vi "Old Master Control Loops.vi"() -> ()   [LabVIEW 2009]
uses:
  lib/DAQ IO/Daq Actions.ctl
  lib/Data Access Objects/Metadata/LBCB Number.ctl
  lib/Control Loop/Parameters Changes.ctl
  lib/Data Access Objects/Metadata/Persistant DAO Actions.ctl
  lib/MixedMode/Mixed Mode States.ctl
  lib/MixedMode/Ramp Time Tuple.ctl
  lib/Data Access Objects/Metadata/LBCB Filter.ctl
  lib/MixedMode/Mixed Mode Command Action.ctl
  lib/MixedMode/Mixed Mode Covergance Status.ctl
  lib/MixedMode/Mixed Mode Cartesian Data.ctl
  lib/MixedMode/Target Data.ctl
  lib/MixedMode/Messages/Mixed Mode Command.ctl
  lib/Data Access Objects/Metadata/LBCB Space.ctl
  lib/Global Data/Cartesian Data type.ctl
  lib/Global Data/Actuator DataType.ctl
  lib/Global Data/Actuator Measurment Actions.ctl
  lib/Global Data/Cartesian Measurment Actions.ctl
  lib/Control Loop/Control Loop State.ctl
  lib/Data Access Objects/Metadata/DAO Actions.ctl
  lib/Control Loop/Parameter Change States.ctl
  lib/MixedMode/Messages/Mixed Mode Status.ctl
  lib/Apps/App Status Actions.ctl
  lib/Logging/LogFileType.ctl
  lib/Launcher/Launcher Actions.ctl
  lib/Launcher/NoPanelAppTypes.ctl
  lib/Autobalance/Autobalance State.ctl
  lib/Apps/Yes No Button.ctl
  lib/Control Loop/Limit Settings.ctl
  lib/Control Loop/Limit Matrix.ctl
  lib/Control Loop/LBCB_Conversions_Actions.ctl
  lib/Data Access Objects/Global Cache/Global Cache.vi
  lib/Data Access Objects/Metadata/LBCB Settings.ctl
  lib/Data Access Objects/Control Loop/PID Controls.ctl
  lib/MixedMode/Stiffness Matrix.ctl
  lib/Data Access Objects/Metadata/LBCB Position.ctl
  lib/Limits/Actuator Faults.ctl
  lib/Limits/Cart Force Faults.ctl
  lib/Limits/Cart Disp Faults.ctl
  lib/Data Access Objects/Metadata/LBCB Size.ctl
  lib/Data Access Objects/Metadata/LBCB Type.ctl
  lib/Control Loop/Act & Cart Measurments.ctl
  lib/Autobalance/Autobalance Status Data.ctl
  lib/Control Loop/Act & Cart Commands.ctl
  lib/Autobalance/Autobalance Stage.ctl
  lib/Autobalance/Autobalance Data Point.ctl
panel:
  in  "Monitor Loop Time":u32
  out "L2 Volts LVDT & LC":dbl[](array[numeric])
  out "L1 Volts LVDT & LC":dbl[](array[numeric])
  out "L2 Autobalance Out":T1[](array[typedef])
  out "L1 Autobalance Out":T1[](array[typedef])
  out "Collecting DAQ Samples":bool
  out "DAQ Volts":dbl[](array[numeric])=[-5.059315779335383, -5.016629198362524, -5.097891313865665, -5.092890991738198, -5.1138932889519, -4.974194835814303, 0.24442110332308561, 0.2508540081873783, -0.00045656932832031883, -0.0010919008583725697, -0.001119467422792373, -0.001138029771633142, 0.051584220664617125, 0.05637080163747566, -0.0007913138656640637, 0.023009008261802286, -0.021593288951899364, 0.0027051641856972383, -5.059665406563526, -5.018353952939143, -5.097893414204858, -5.0928919356893525, -5.11389113151188, -4.974191443340161, 0.24267296718237016, 0.2422302353042843, -0.0004670710242903981, -0.0011032282722249686, -0.0010935781425555466, -0.0010973200819313358, 0.05123459343647403, 0.05464604706085686, -0.0007934142048580796, 0.02300806431064792, -0.02159113151187963, 0.0027085566598390553, 0.048884220664617124, 0.04853459343647403, 0.050170801637475664, 0.04844604706085686, -9.131386566406377e-05, -9.341420485807962e-05]
  in  "Volt Logger Time":u32
  out "All Stopped":bool
  out "L2 Previous Target":T5
  out "L1 Previous Target":T5
  out "L2 Iterative Target":T6
  out "L1 Iterative Target":T6
  out "Mixed Mode":i32
  out "Status Changes":i32
  out "L2 Control Rate":i32
  out "DAQ Started":bool
  out "L2 Current Target":T6
  out "L1 Current Target":T6
  out "Logging Directory":path
  out "L2 Auto Balance Error Tolerance":dbl[](array[numeric])=[0.01, 0.01, 0.01, 0.01, 0.01, 0.01]
  out "L1 Auto Balance Error Tolerance":dbl[](array[numeric])=[0.01, 0.01, 0.01, 0.01, 0.01, 0.01]
  out "L2 PID Control":T8={"I-Control"=TRUE, "Ctrl Mode"=TRUE}
  in  "Hold Period":bool
  in  "Averaging":bool
  out "L1 Ctrl Loop State":T9
  out "L2 Max Increment":dbl[](array[numeric])
  out "L2 Jacobian Gain":dbl[](array[numeric])
  out "L2 Force Error Range":dbl[](array[numeric])
  out "L1 Max Increment":dbl[](array[numeric])
  out "L1 Jacobian Gain":dbl[](array[numeric])
  out "L1 Force Error Range":dbl[](array[numeric])
  out "L2 Commands":T10
  out "L1 Commands":T10
  out "L2 I Gain":dbl[](array[numeric])=[0.3, 0.3, 0.3, 0.3, 0.3, 0.3]
  in  "L2 PID On":bool
  in  "L2 Faults":T14
  in  "L2 Ctrl Loop In Actuator":dbl[](array[numeric])
  out "L2 Cmd  Volts":dbl[](array[numeric])
  out "L2 Ctrl Loop Out Actuator":dbl[](array[numeric])=[0.012801822908652838, 0.012801822908652838, 7.98290599846041e-06, 8.154359441903125e-06, 8.154359441903125e-06, 8.154359441903125e-06]
  out "L2 P Gain":dbl[](array[numeric])
  out "L2 I Const":dbl[](array[numeric])
  in  "Ramp Time":u32
  out "LBCB 2 Setting":T15={"Size"=enum."1/5th-scale LBCB", "Type"=enum."Left Hand Type"}
  out "L2 Limits":T18
  out "L1  Limits":T18
  out "L2 Position":T20={"Motion Center"=[0.0, 0.0, 0.0], "Transformation Matrix"=[[1.0, 0.0, 0.0, 0.0, 0.0, 0.0], [0.0, 1.0, 0.0, 0.0, 0.0, 0.0], [0.0, 0.0, 1.0, 0.0, 0.0, 0.0], [0.0, 0.0, 0.0, 1.0, 0.0, 0.0], [0.0, 0.0, 0.0, 0.0, 1.0, 0.0], [0.0, 0.0, 0.0, 0.0, 0.0, 1.0]]}
  out "L1  Position":T20={"Motion Center"=[0.0, 0.0, 0.0], "Transformation Matrix"=[[1.0, 0.0, 0.0, 0.0, 0.0, 0.0], [0.0, 1.0, 0.0, 0.0, 0.0, 0.0], [0.0, 0.0, 1.0, 0.0, 0.0, 0.0], [0.0, 0.0, 0.0, 1.0, 0.0, 0.0], [0.0, 0.0, 0.0, 0.0, 1.0, 0.0], [0.0, 0.0, 0.0, 0.0, 0.0, 1.0]]}
  out "L1 Measurements":T21
  out "L2 Measurements":T21
  out "L1 Stiffness Jacobian":T22=[[1000000.0, 0.0, 0.0, 0.0, 0.0, 0.0], [0.0, 1000000.0, 0.0, 0.0, 0.0, 0.0], [0.0, 0.0, 1000000.0, 0.0, 0.0, 0.0], [0.0, 0.0, 0.0, 1000000.0, 0.0, 0.0], [0.0, 0.0, 0.0, 0.0, 1000000.0, 0.0], [0.0, 0.0, 0.0, 0.0, 0.0, 1000000.0]]
  out "L2 Stiffness Jacobian":T22=[[1000000.0, 0.0, 0.0, 0.0, 0.0, 0.0], [0.0, 1000000.0, 0.0, 0.0, 0.0, 0.0], [0.0, 0.0, 1000000.0, 0.0, 0.0, 0.0], [0.0, 0.0, 0.0, 1000000.0, 0.0, 0.0], [0.0, 0.0, 0.0, 0.0, 1000000.0, 0.0], [0.0, 0.0, 0.0, 0.0, 0.0, 1000000.0]]
  out "L1 Convergence Status":T23
  out "L2 Convergence Status":T23
  out "MixedModeStates":T24
  out "L1 PID Control":T8={"I-Control"=TRUE, "Ctrl Mode"=TRUE}
  in  "L1 PID On":bool
  in  "L1 Faults":T14
  out "L1 P Gain":dbl[](array[numeric])
  out "L1 I Gain":dbl[](array[numeric])=[0.3, 0.3, 0.3, 0.3, 0.3, 0.3]
  out "L1 I Const":dbl[](array[numeric])
  out "LBCB 1 Control Loop Force Limit":bool
  out "LBCB 1 Setting":T15={"Size"=enum."1/5th-scale LBCB", "Type"=enum."Left Hand Type"}
  out "L2 Ctrl Loop State":T9
  out "L1 Cmd  Volts":dbl[](array[numeric])
  out "L1 Ctrl Loop Out Actuator":dbl[](array[numeric])=[0.012801822908652838, 0.012801822908652838, 7.98290599846041e-06, 8.154359441903125e-06, 8.154359441903125e-06, 8.154359441903125e-06]
  out "L1 Control Rate":i32=50 caption="Control Rate"
  in  "L1 Ctrl Loop In Actuator":dbl[](array[numeric])
  out "L2 Servo Error":dbl[](array[numeric])=[-0.014471871278962644, -0.0027477897622864888, 0.03594582291831433, -0.006177356244415369, -0.000527948512754489, 0.04718526152757189]
  out "L2 Actuator Meas. Disp & Forces":dbl[](array[numeric])=[0.015224103858920254, 0.016374115079328375, 0.0001743188568230551, 0.03971045114557009, 0.007082336209989981, 0.009859079687370698, 8.685887933911959, 1.9897804119684945, 4.857688782335148, 93.30834661628205, -5.911514458784602, -1.446477360303783]
  out "Number of \nExternal \nChannels":i32
  out "DAQ Enabled":bool
  in  "App Running":bool
  out "DAQ Rate":i32=2 caption="Control Rate"
  out "L1 Servo Error":dbl[](array[numeric])=[-0.014471871278962644, -0.0027477897622864888, 0.03594582291831433, -0.006177356244415369, -0.000527948512754489, 0.04718526152757189]
  out "L1 Actuator Meas. Disp & Forces":dbl[](array[numeric])=[0.015224103858920254, 0.016374115079328375, 0.0001743188568230551, 0.03971045114557009, 0.007082336209989981, 0.009859079687370698, 8.685887933911959, 1.9897804119684945, 4.857688782335148, 93.30834661628205, -5.911514458784602, -1.446477360303783]
  out "External Sensors":dbl[](array[numeric])
  out "DAQ Overflow":bool
  # "Cmd"
  # "Servo"
  # "Cmd"
  # "Servo"
  # "Cmd"
  # "Servo"
  # "Cmd"
  # "Servo"
  # "Continuous"
  # "Hold"
  # "(inch)"
  # "X"
  # "(inch)"
  # "Y"
  # "(inch)"
  # "Z"
  # "Xglobal = T*Xlocal"
  # "(inch)"
  # "X"
  # "(inch)"
  # "Y"
  # "(inch)"
  # "Z"
  # "Xglobal = T*Xlocal"
  # "Continuous"
  # "Hold"
types:
  T1 = typedef "Autobalance Status Data.ctl" = cluster{"IsBalanced":T2, "Autobalance Stage":T3, "High":T4, "Low":T4, "Balanced \nCmd":dbl}
  T2 = typedef "Yes No Button.ctl" = bool
  T3 = typedef "Autobalance Stage.ctl" = enum16{"Coarse", "Fine", "Backing Up", "Done"}
  T4 = typedef "Autobalance Data Point.ctl" = cluster{"cCmd":dbl, "cServo":dbl, "pCmd":dbl, "pServo":dbl}
  T5 = typedef "Mixed Mode Cartesian Data.ctl" = cluster{"Displacements":dbl[], "Forces":dbl[]}
  T6 = typedef "Target Data.ctl" = cluster{"Displacements":dbl[], "Command Type":enum16{"<None>", "Displacement", "Force"}[], "Forces":dbl[], "Space":T7}
  T7 = typedef "LBCB Space.ctl" = enum16{"Actuator", "Cartesian"}
  T8 = typedef "PID Controls.ctl" = cluster{"I-Control":bool, "Ctrl Mode":bool}
  T9 = typedef "Control Loop State.ctl" = enum16{"Idle", "Off", "Reset Autobalancing", "Autobalancing", "Set Command", "Ready for Control", "On"}
  T10 = typedef "Act & Cart Commands.ctl" = cluster{"Act Cmd":dbl[], "Cart Cmd":dbl[]}
  T11 = typedef "Actuator Faults.ctl" = cluster{"X1":bool, "X2":bool, "Y1":bool, "Z1":bool, "Z2":bool, "Z3":bool}
  T12 = typedef "Cart Force Faults.ctl" = cluster{"Fx":bool, "Fy":bool, "Fz":bool, "Mx":bool, "My":bool, "Mz":bool}
  T13 = typedef "Cart Disp Faults.ctl" = cluster{"Dx":bool, "Dy":bool, "Dz":bool, "Rx":bool, "Ry":bool, "Rz":bool}
  T14 = cluster{"Act Disp":T11, "Act Force":T11, "Cart Force":T12, "Cart Disp":T13}
  T15 = typedef "LBCB Settings.ctl" = cluster{"Size":T16, "Type":T17}
  T16 = typedef "LBCB Size.ctl" = enum16{"1/5th-scale LBCB", "Full-scale LBCB", "Portable LBCB"}
  T17 = typedef "LBCB Type.ctl" = enum16{"Right Hand Type", "Left Hand Type"}
  T18 = typedef "Limit Settings.ctl" = cluster{"Actuator Force Limits":T19, "Actuator Stroke Limits":T19, "Cartesian Disp Limit":T19, "Cartesian Force Limit":T19, "Command Voltage Limit":T19}
  T19 = typedef "Limit Matrix.ctl" = dbl[][]
  T20 = typedef "LBCB Position.ctl" = cluster{"Motion Center":dbl[], "Transformation Matrix":dbl[][]}
  T21 = typedef "Act & Cart Measurments.ctl" = cluster{"Act Disp":dbl[], "Act Forces":dbl[], "Cart Disp":dbl[], "Cart Forces":dbl[]}
  T22 = typedef "Stiffness Matrix.ctl" = dbl[][]
  T23 = typedef "Mixed Mode Covergance Status.ctl" = cluster{"IsConverged":bool[], "Force Errors":dbl[], "MaxForceDiffIndex":i32}
  T24 = typedef "Mixed Mode States.ctl" = enum16{"Init", "Wait For DAQ", "Idle", "Start Initial Position", "Initial Position", "Start Initial Ramp", "Run Initial Ramp", "Start Iterative Stage", "Convergence Check", "Update Stiffness Jacobian", "Update Command", "Start Iterative Ramp", "Run Iterative Ramp", "Start Iterative Stabilize", "Iterative Stabilize", "Start Iterative Holding", "Iterative Holding", "Start Stabilize", "Stabilize", "Start Hold", "Holding", "Done", "Aborting", "Exit", "Nop"}
  T25 = typedef "Persistant DAO Actions.ctl" = enum16{"Init", "Get", "Set", "Load", "Save"}
  T26 = typedef "Autobalance State.ctl" = enum16{"Init", "Send High ", "Wait High", "Read High Start", "Read High", "Send Low", "Wait Low", "Read Low Start", "Read Low", "Publish", "Calculate", "Done"}
  T27 = typedef "Ramp Time Tuple.ctl" = cluster{"Ramp":dbl, "Stab":dbl, "Hold":dbl}
  T28 = typedef "Mixed Mode Command Action.ctl" = enum16{"Start Command", "Stop", "Exit", "No Op", "Start Acquisition", "Measure Initial Position"}
  T29 = typedef "LBCB Number.ctl" = enum16{"LBCB1", "LBCB2"}
  T30 = typedef "Mixed Mode Status.ctl" = cluster{"LBCB Target":T6[], "MixedModeStates":T24, "LBCB Convergence":T23[], "LBCB Measurements":T5[]}
  T31 = typedef "Mixed Mode Command.ctl" = cluster{"Command":T28, "Ramp Times":cluster{"Initial":T27, "Iterative":T27}, "LBCB1":T6, "LBCB2":T6}
  T32 = typedef "Parameters Changes.ctl" = cluster{"Change State":T33, "LBCB Number":T29}
  T33 = typedef "Parameter Change States.ctl" = enum16{"Mixed Mode", "Control Loop", "Limits", "Application", "Stiffness Jacobian", "Start DAQ", "Auto-Balancing", "Set Command", "Enable Control", "Disable Control", "Stop Application"}
  T34 = typedef "Cartesian Point.ctl" = cluster{"Dx":dbl, "Dy":dbl, "Dz":dbl, "Rx":dbl, "Ry":dbl, "Rz":dbl}
  T35 = typedef "Actuator Matrix.ctl" = cluster{"Lower":T36, "Upper":T36}
  T36 = typedef "Actuator Point.ctl" = cluster{"X1":dbl, "X2":dbl, "Y1":dbl, "Z1":dbl, "Z2":dbl, "Z3":dbl}
  T37 = typedef "Cartesian Matrix.ctl" = cluster{"Lower":T34, "Upper":T34}
  T38 = typedef "App Parameters.ctl" = cluster{"Monitor Loop":T39, "Ramp Time":T39, "Log Loop":T39, "TCP to DAQ":T39, "Logging Directory":path, "Log File Size (MBytes)":i64, "Volt Logging Loop":T39}
  T39 = typedef "Timing Parameters.ctl" = cluster{"Interval":dbl, "Rate ":dbl}
  T40 = typedef "Number Of LBCBs.ctl" = enum16{"1", "2"}
  T41 = typedef "DAO Actions.ctl" = enum16{"Init", "Get", "Set"}
  T42 = typedef "Actuator Measurment Actions.ctl" = enum16{"Set  Data", "Get", "Init"}
  T43 = typedef "Actuator DataType.ctl" = cluster{"LVDTs":dbl[], " Commands":dbl[], "Load Cells":dbl[], "Servo":dbl[]}
  T44 = typedef "Cartesian Data type.ctl" = cluster{"Displacements":dbl[], "Forces":dbl[], "Displacement Commands":dbl[]}
  T45 = typedef "Cartesian Measurment Actions.ctl" = enum16{"Set Data", "Get", "Init", "Set Offsets"}
  T46 = typedef "Calibration Settings.ctl" = cluster{"Command Sensitivity":dbl[], "Servo Error Offset":dbl[], "LVDT Sensitivity":dbl[], "LVDT Offset":dbl[], "Load Cell Offsets":dbl[], "Load Cell Sensitivity":dbl[]}
  T47 = typedef "Autobalance Control Parameters.ctl" = cluster{"Number of Samples":i32, "Delay After Cmd":i32, "Maximum Command":dbl}
  T48 = typedef "App Status Actions.ctl" = enum16{"Init", "Get Status", "Running", "Control", "Autobalanced", "Data Acquisition", "Set App State", "DAQ Started", "Set LBCB State", "Set All", "Set Cont Logging", "Set Step Logging", "Set MM Logging", "Set Volt Logging", "Set Cart Type", "Set DAQ Link", "Set NTCP Link"}
  T49 = typedef "Ramp Time Input.ctl" = cluster{"Directional":T50, "Iterative":T50}
  T50 = typedef "Ramp Control.ctl" = cluster{"Ramp":dbl, "Stabilize":dbl, "Hold":dbl}
  T51 = typedef "App Status.ctl" = cluster{"Running":bool, "Controlling L2":bool, "Autobalance L2":bool, "Data Acquisition":bool, " App State":T52, "DAQ Started":bool, "LBCB 1 State":T53, "LBCB 2 State":T53, "Controlling L1":bool, "Autobalance L1":bool, "Cartesian Type":bool, "Continuous Logging":bool, "Step Logging":bool, "Voltage Logging":bool, "Mixed Mode Logging":bool, "DAQ Link":bool, "NTCP Link ":bool}
  T52 = typedef "AppStates.ctl" = enum16{"Starting OM", "Initializing Displays", "Setting up Archiving", "Setting Up DAQ Channels", "Start DAQ", "DAQ Starting", "Controlling LBCBs", "Stopping OM"}
  T53 = typedef "Lbcb Control Loop States.ctl" = enum16{"Idle", "Start Selected", "Load Last Command", "Start Autobalancing", "Autobalancing", "Control Loop Initialized", "Control Enabled"}
  T54 = typedef "LBCB_Conversions_Actions.ctl" = enum16{"A2C", "C2A", "Set Log Filename", "Init"}
  T55 = cluster{"Act Disp":dbl[], "Act Forces":dbl[], "Cart Disp":dbl[], "Cart Forces":dbl[]}
  T56 = typedef "Measurements.ctl" = cluster{"Act Disp":dbl[], "Act Forces":dbl[], "Cart Disp":dbl[], "Cart Forces":dbl[]}
  T57 = typedef "Daq Actions.ctl" = enum16{"Init", "Send Commands", "Get Responses", "Stop"}
  T58 = enum16{"open", "replace", "create", "open or create", "replace or create", "replace or create with confirmation"}
  T59 = typedef "LogFileType.ctl" = enum16{"Continuous", "Step", "Volts", "Offsets", "Mixed Mode State", "DLL  Errors", "End List"}
  T60 = typedef "LBCB Filter.ctl" = enum16{"LBCB 1", "LBCB 2", "Both"}
  T61 = typedef "NoPanelAppTypes.ctl" = enum16{"NTCP Socket", "Data Archiving", "DAQ Link", "Control Loops", "Autobalance Monitor", "Mixed Mode Monitor", "Cmd Disp Diffs"}
  T62 = typedef "Launcher Actions.ctl" = enum16{"Launch", "Stop All", "Stop", "Kill", "Running?", "Init"}
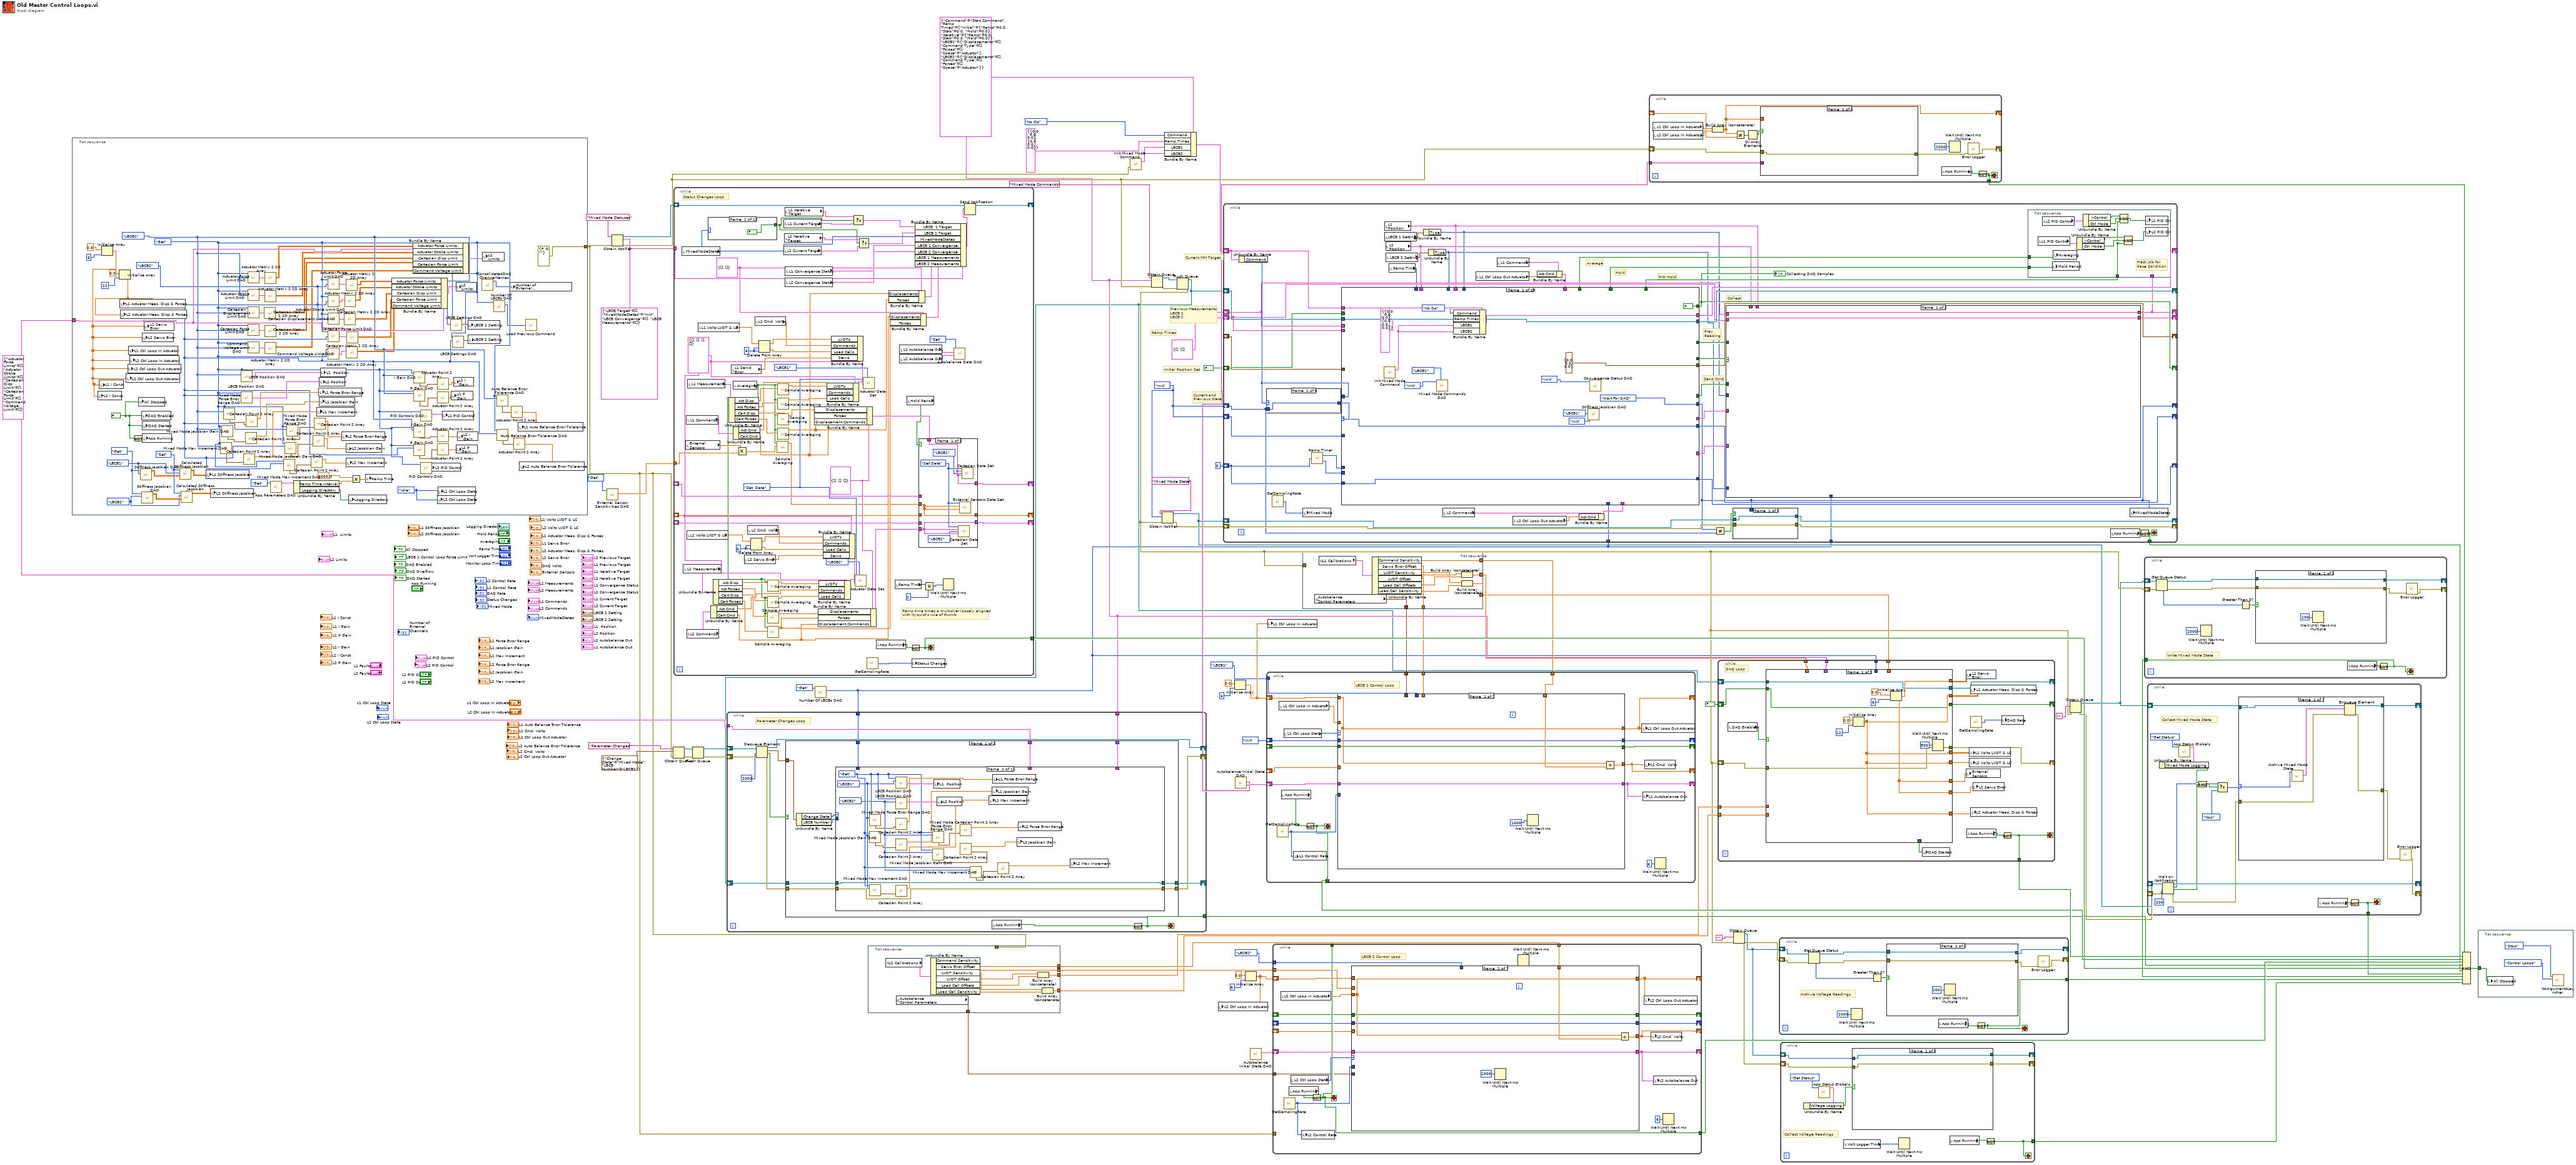
[diagram p0: block diagram]
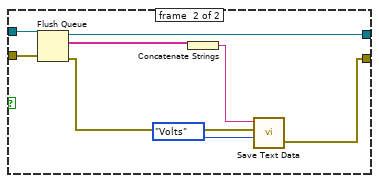
[diagram p2: hidden frame]
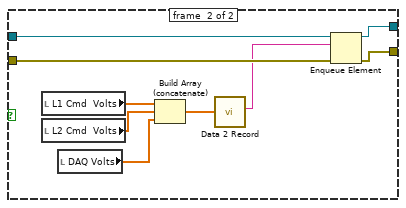
[diagram p3: hidden frame]
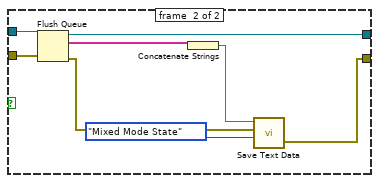
[diagram p4: hidden frame]
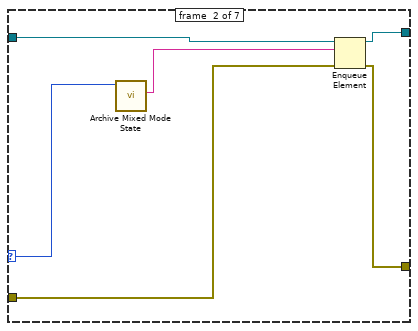
[diagram p5: hidden frame]
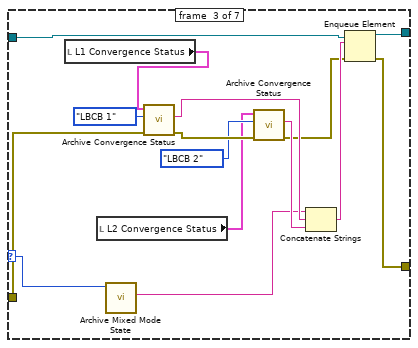
[diagram p6: hidden frame]
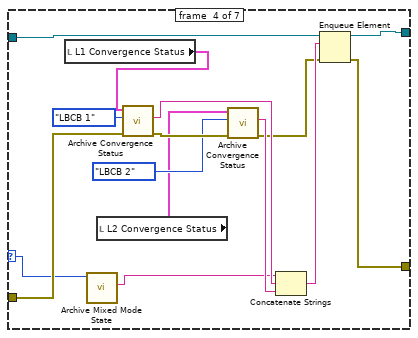
[diagram p7: hidden frame]
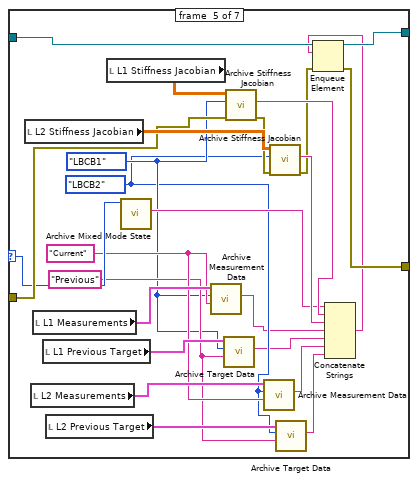
[diagram p8: hidden frame]
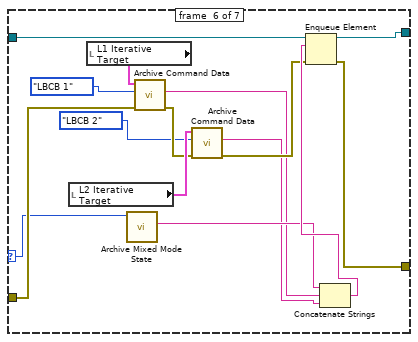
[diagram p9: hidden frame]
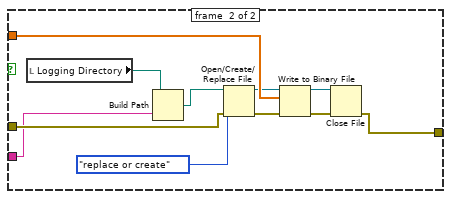
[diagram p11: hidden frame]
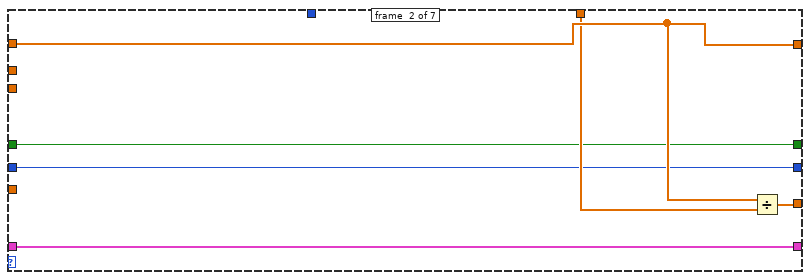
[diagram p12: hidden frame]
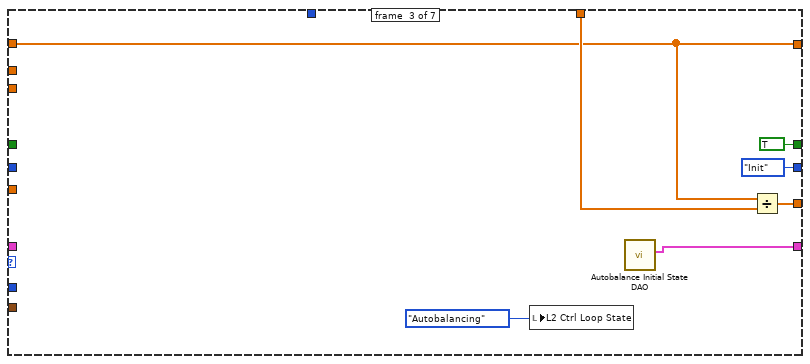
[diagram p13: hidden frame]
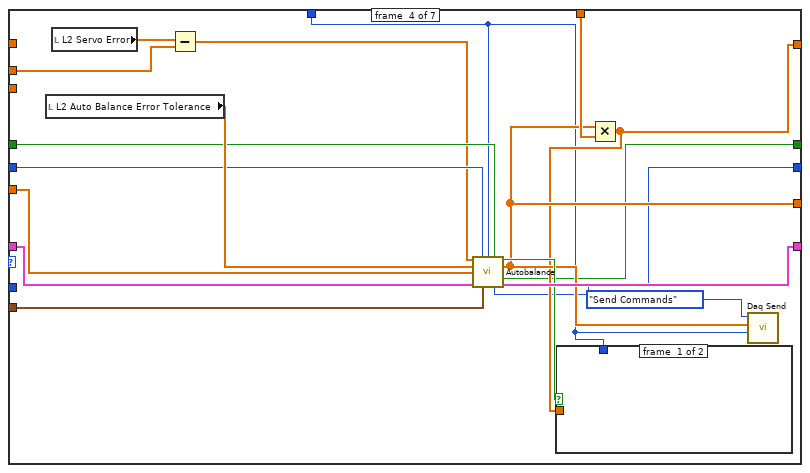
[diagram p14: hidden frame]
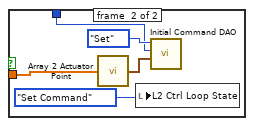
[diagram p15: hidden frame]
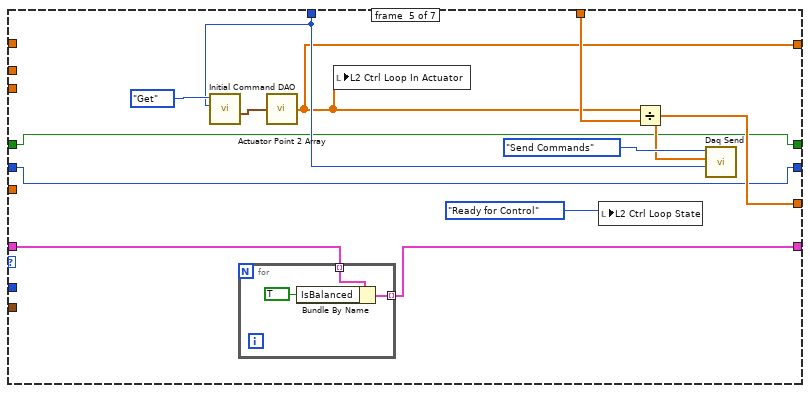
[diagram p16: hidden frame]
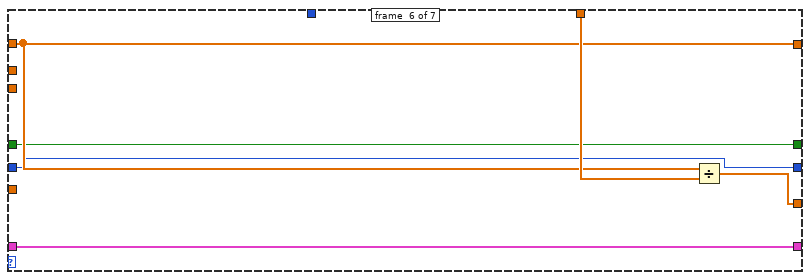
[diagram p17: hidden frame]
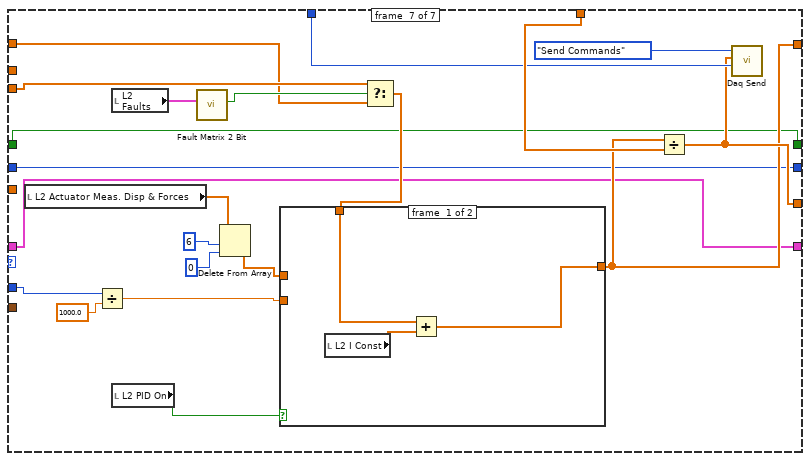
[diagram p18: hidden frame]
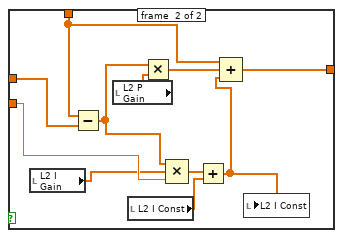
[diagram p19: hidden frame]
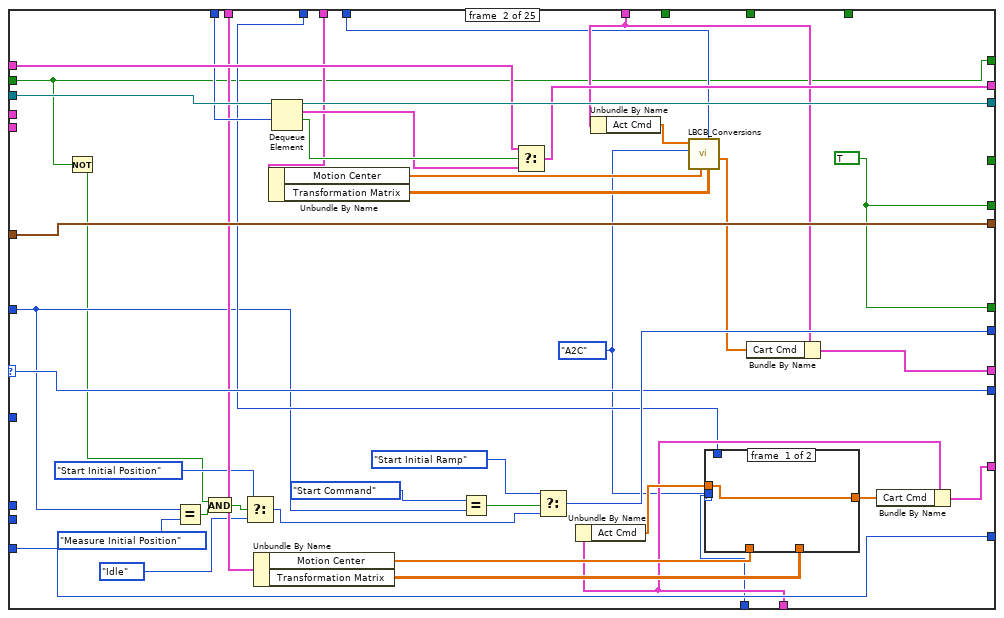
[diagram p20: hidden frame]
diagram:
  w9 = T18 {"Actuator Force Limits"=[], "Actuator Stroke Limits"=[], "Cartesian Disp Limit"=[], "Cartesian Force Limit"=[], "Command Voltage Limit"=[]} ("L1  Limits")
  w60 = T30 {"LBCB Target"=[], "MixedModeStates"=enum."Init", "LBCB Convergence"=[], "LBCB Measurements"=[]} ("Mixed Mode Status")
  w66 = T5 {"Displacements"=[], "Forces"=[]} ("Cartesian  Data")
  w3 = T31 {"Command"=enum."Start Command", "Ramp Times"={"Initial"={"Ramp"=0.0, "Stab"=0.0, "Hold"=0.0}, "Iterative"={"Ramp"=0.0, "Stab"=0.0, "Hold"=0.0}}, "LBCB1"={"Displacements"=[], "Command Type"=[], "Forces"=[], "Space"=enum."Actuator"}, "LBCB2"={"Displacements"=[], "Command Type"=[], "Forces"=[], "Space"=enum."Actuator"}} ("Mixed Mode Command")
  w70 = Mixed_Mode_States."Init" ("MixedModeStates")
  # "Initial Position Set"
  # "Current MM Target"
  # "Current and\nPrevious State"
  # "Previous Measurements\nLBCB 1\nLBCB 2"
  # "Ramp Times"
  n1 = flat-sequence {
    tunnel: [errorcluster {"status"=FALSE, "code"=0, "source"=""} ("error out")] -> w13
    tunnel: w9 -> [w95]
    frame #0 {
      w103 = Control_Loop_State."Idle" ("L1 Ctrl Loop State")
      w98 = LBCB_Number."LBCB2" ("ID")
      w100 = LBCB_Number."LBCB1" ("ID")
      w99 = Persistant_DAO_Actions."Get" ("Actuator Force Limit Actions")
      w112 = FALSE
      w138 = Persistant_DAO_Actions."Set" ("Actions")
      w135 = LBCB_Number."LBCB1" ("LBCB Number")
      w136 = LBCB_Number."LBCB2" ("LBCB Number")
      w134 = Persistant_DAO_Actions."Get" ("Actions")
      n2 = Initialize Array(0.0 ("element"), 6 ("dimension size")) -> (w102:dbl[])
      n3 = local write "L2 I Const"(w102) -> ()
      n4 = local write "L1 I Const"(w102) -> ()
      n5 = Initialize Array(0.0 ("element"), 12 ("dimension size")) -> (w104:dbl[])
      n6 = local write "L1 Actuator Meas. Disp & Forces"(w104) -> ()
      n7 = local write "L2 Actuator Meas. Disp & Forces"(w104) -> ()
      n8 = local write "L2 Ctrl Loop Out Actuator"(w102) -> ()
      n9 = local write "L1 Ctrl Loop Out Actuator"(w102) -> ()
      n10 = local write "L1 Ctrl Loop In Actuator"(w102) -> ()
      n11 = local write "L2 Ctrl Loop In Actuator"(w102) -> ()
      n12 = Not(x=w112) -> (.not. x?=w131:bool)
      n13 = local write "All Stopped"(w112) -> ()
      n14 = call "Stiffness Jacobian DAO.vi"("LBCB Number"=w135, "Actions"=w134) -> ("Stiffness Jacobian Out"=w137:T22)  [unwired: 3 in, 6 out]
      n15 = local write "DAQ Enabled"(w112) -> ()
      n16 = call "Stiffness Jacobian DAO.vi"("LBCB Number"=w136, "Actions"=w134) -> ("Stiffness Jacobian Out"=w139:T22)  [unwired: 3 in, 6 out]
      n17 = local write "L2 Servo Error"(w102) -> ()
      n18 = local write "DAQ Started"(w112) -> ()
      n19 = local write "App Running"(w131) -> ()
      n20 = local write "L1 Servo Error"(w102) -> ()
      n21 = call "Calculated Stiffness Jacobian.vi"("Stiffness Jacobian In"=w137, "LBCB Number"=w135, "Actions"=w138) -> ("Stiffness Jacobian Out"=w132:T22)  [unwired: 1 in, 7 out]
      n22 = call "Calculated Stiffness Jacobian.vi"("Stiffness Jacobian In"=w139, "LBCB Number"=w136, "Actions"=w138) -> ("Stiffness Jacobian Out"=w133:T22)  [unwired: 1 in, 7 out]
      n23 = local write "L1 Stiffness Jacobian"(w132) -> ()
      n24 = local write "L2 Stiffness Jacobian"(w133) -> ()
      n25 = call "Mixed Mode Max Increment DAO.vi"("Max Increment Actions"=w99, "LBCB Number"=w100) -> ("Max Increment Out"=w150:T34)  [unwired: 3 in, 10 out]
      n26 = call "Mixed Mode Jacobian Gain DAO.vi"("Jacobian Gain Actions"=w99, "LBCB Number"=w100) -> ("Jacobian Gain Out"=w149:T34)  [unwired: 3 in, 10 out]
      n27 = call "Mixed Mode Force Error Range DAO.vi"("Force Error Range Actions"=w99, "LBCB Number"=w100) -> ("Force Error Range Out"=w148:T34)  [unwired: 3 in, 10 out]
      n28 = call "LBCB Position DAO.vi"("LBCB Settings Actions"=w99, "LBCB Number"=w100) -> ("LBCB Position Output"=w147:T20)  [unwired: 3 in, 10 out]
      n29 = call "LBCB Position DAO.vi"("LBCB Settings Actions"=w99, "LBCB Number"=w98) -> ("LBCB Position Output"=w146:T20)  [unwired: 3 in, 10 out]
      n30 = call "Cartesian Point 2 Array.vi"("Cart Disp"=w150) -> ("Array"=w143:dbl[])  [unwired: 2 out]
      n31 = call "Cartesian Point 2 Array.vi"("Cart Disp"=w149) -> ("Array"=w144:dbl[])  [unwired: 2 out]
      n32 = call "Cartesian Point 2 Array.vi"("Cart Disp"=w148) -> ("Array"=w145:dbl[])  [unwired: 2 out]
      n33 = call "Actuator Force Limit DAO.vi"("Actuator Force Limit Actions"=w99, "ID"=w100) -> ("Actuator Force Limits Out"=w94:T35)  [unwired: 3 in, 10 out]
      n34 = call "Actuator Stroke Limit DAO.vi"("Actuator Stroke Limit Actions"=w99, "ID"=w100) -> ("Actuator Stroke Limits Out"=w93:T35)  [unwired: 3 in, 10 out]
      n35 = call "Cartesian Displacement Limit DAO.vi"("Cartesian Displacement Limit Actions"=w99, "ID"=w100) -> ("Cartesian Displacement Out"=w88:T37)  [unwired: 3 in, 10 out]
      n36 = call "Cartesian Force Limit DAO.vi"("Cartesian Force Limit Actions"=w99, "ID"=w100) -> ("Cartesian Force Limit Out"=w87:T37)  [unwired: 3 in, 10 out]
      n37 = call "Command Voltage Limit DAO.vi"("Actuator Stroke Limit Actions"=w99, "ID"=w100) -> ("Command Voltage Limit Out"=w92:T35)  [unwired: 3 in, 10 out]
      n38 = call "Cartesian Matrix 2 2D Array.vi"("Matrix In"=w88) -> ("Matrix Out"=w76:T19)  [unwired: 10 out]
      n39 = call "Actuator Matrix 2 2D Array.vi"("Matrix In"=w94) -> ("Matrix Out"=w91:T19)  [unwired: 10 out]
      n40 = call "Actuator Matrix 2 2D Array.vi"("Matrix In"=w93) -> ("Matrix Out"=w90:T19)  [unwired: 10 out]
      n41 = call "Cartesian Matrix 2 2D Array.vi"("Matrix In"=w87) -> ("Matrix Out"=w75:T19)  [unwired: 10 out]
      n42 = call "Actuator Matrix 2 2D Array.vi"("Matrix In"=w92) -> ("Matrix Out"=w89:T19)  [unwired: 10 out]
      n43 = call "App Parameters DAO.vi"("Actions"=Persistant_DAO_Actions."Get") -> ("Application Timing and Logging Out"=w154:T38)  [unwired: 3 in, 7 out]
      n44 = call "Mixed Mode Max Increment DAO.vi"("Max Increment Actions"=w99, "LBCB Number"=w98) -> ("Max Increment Out"=w111:T34)  [unwired: 3 in, 10 out]
      n45 = call "Mixed Mode Jacobian Gain DAO.vi"("Jacobian Gain Actions"=w99, "LBCB Number"=w98) -> ("Jacobian Gain Out"=w110:T34)  [unwired: 3 in, 10 out]
      n46 = call "Mixed Mode Force Error Range DAO.vi"("Force Error Range Actions"=w99, "LBCB Number"=w98) -> ("Force Error Range Out"=w109:T34)  [unwired: 3 in, 10 out]
      n47 = Unbundle By Name(w154) -> ("Ramp Time.Interval"=w155:dbl, "Logging Directory"=w151:path)
      n48 = call "Cartesian Point 2 Array.vi"("Cart Disp"=w111) -> ("Array"=w140:dbl[])  [unwired: 1 in, 1 out]
      n49 = call "Cartesian Point 2 Array.vi"("Cart Disp"=w110) -> ("Array"=w141:dbl[])  [unwired: 1 in, 1 out]
      n50 = call "Cartesian Point 2 Array.vi"("Cart Disp"=w109) -> ("Array"=w142:dbl[])  [unwired: 1 in, 1 out]
      n51 = local write "L1 Max Increment"(w143) -> ()
      n52 = local write "L1 Force Error Range"(w145) -> ()
      n53 = local write "L1 Jacobian Gain"(w144) -> ()
      n54 = local write "L2 Position"(w146) -> ()
      n55 = local write "L1  Position"(w147) -> ()
      n56 = call "Actuator Force Limit DAO.vi"("Actuator Force Limit Actions"=w99, "ID"=w98) -> ("Actuator Force Limits Out"=w86:T35)  [unwired: 3 in, 10 out]
      n57 = call "Actuator Stroke Limit DAO.vi"("Actuator Stroke Limit Actions"=w99, "ID"=w98) -> ("Actuator Stroke Limits Out"=w85:T35)  [unwired: 3 in, 10 out]
      n58 = call "Cartesian Displacement Limit DAO.vi"("Cartesian Displacement Limit Actions"=w99, "ID"=w98) -> ("Cartesian Displacement Out"=w84:T37)  [unwired: 3 in, 10 out]
      n59 = call "Cartesian Force Limit DAO.vi"("Cartesian Force Limit Actions"=w99, "ID"=w98) -> ("Cartesian Force Limit Out"=w83:T37)  [unwired: 3 in, 10 out]
      n60 = call "Command Voltage Limit DAO.vi"("Actuator Stroke Limit Actions"=w99, "ID"=w98) -> ("Command Voltage Limit Out"=w82:T35)  [unwired: 3 in, 10 out]
      n61 = local write "L2 Force Error Range"(w142) -> ()
      n62 = call "Cartesian Matrix 2 2D Array.vi"("Matrix In"=w84) -> ("Matrix Out"=w79:T19)  [unwired: 10 out]
      n63 = call "Actuator Matrix 2 2D Array.vi"("Matrix In"=w85) -> ("Matrix Out"=w80:T19)  [unwired: 10 out]
      n64 = local write "L2 Jacobian Gain"(w141) -> ()
      n65 = call "Actuator Matrix 2 2D Array.vi"("Matrix In"=w86) -> ("Matrix Out"=w81:T19)  [unwired: 10 out]
      n66 = call "Actuator Matrix 2 2D Array.vi"("Matrix In"=w82) -> ("Matrix Out"=w77:T19)  [unwired: 10 out]
      n67 = local write "L2 Max Increment"(w140) -> ()
      n68 = call "Cartesian Matrix 2 2D Array.vi"("Matrix In"=w83) -> ("Matrix Out"=w78:T19)  [unwired: 10 out]
      n69 = local write "Logging Directory"(w151) -> ()
      n70 = Multiply(x=1000.0, y=w155) -> (x*y=w152:dbl)
      n71 = local write "Ramp Time"(w152) -> ()
      n72 = Bundle By Name(cluster=w95, "Actuator Force Limits"=w81, "Actuator Stroke Limits"=w80, "Cartesian Disp Limit"=w79, "Cartesian Force Limit"=w78, "Command Voltage Limit"=w77) -> (w96:T18)
      n73 = Bundle By Name(cluster=w95, "Actuator Force Limits"=w91, "Actuator Stroke Limits"=w90, "Cartesian Disp Limit"=w76, "Cartesian Force Limit"=w75, "Command Voltage Limit"=w89) -> (w97:T18)
      n74 = call "I Gain DAO.vi"("I Gain Actions"=w99, "LBCB Number"=w100) -> ("I Gain"=w127:T36)  [unwired: 3 in, 10 out]
      n75 = call "P Gain DAO.vi"("P Gain Actions"=w99, "LBCB Number"=w100) -> ("P Gain"=w128:T36)  [unwired: 3 in, 10 out]
      n76 = call "I Gain DAO.vi"("I Gain Actions"=w99, "LBCB Number"=w98) -> ("I Gain"=w130:T36)  [unwired: 3 in, 10 out]
      n77 = call "P Gain DAO.vi"("P Gain Actions"=w99, "LBCB Number"=w98) -> ("P Gain"=w129:T36)  [unwired: 3 in, 10 out]
      n78 = call "PID Controls DAO.vi"("Actions"=w99) -> ("PID Control  Out"=w125:T8)  [unwired: 3 in, 7 out]
      n79 = call "PID Controls DAO.vi"("Actions"=w99) -> ("PID Control  Out"=w126:T8)  [unwired: 3 in, 7 out]
      n80 = local write "L2 PID Control"(w125) -> ()
      n81 = call "Actuator Point 2 Array.vi"("Actuator Point"=w127) -> ("Array"=w124:dbl[])
      n82 = call "Actuator Point 2 Array.vi"("Actuator Point"=w128) -> ("Array"=w123:dbl[])
      n83 = call "Actuator Point 2 Array.vi"("Actuator Point"=w130) -> ("Array"=w122:dbl[])
      n84 = call "Actuator Point 2 Array.vi"("Actuator Point"=w129) -> ("Array"=w121:dbl[])
      n85 = local write "L2 Ctrl Loop State"(w103) -> ()
      n86 = local write "L1 Ctrl Loop State"(w103) -> ()
      n87 = local write "L1 PID Control"(w126) -> ()
      n88 = call "LBCB Settings DAO.vi"("LBCB Number"=w100, "Actions"=w99) -> ("LBCB Setting Out"=w119:T15)  [unwired: 3 in, 6 out]
      n89 = local write "L1 P Gain"(w123) -> ()
      n90 = call "LBCB Settings DAO.vi"("LBCB Number"=w98, "Actions"=w99) -> ("LBCB Setting Out"=w118:T15)  [unwired: 3 in, 6 out]
      n91 = local write "L1 I Gain"(w124) -> ()
      n92 = local write "L2 Limits"(w96) -> ()
      n93 = local write "L2 P Gain"(w121) -> ()
      n94 = local write "L2 I Gain"(w122) -> ()
      n95 = local write "LBCB 1 Setting"(w119) -> ()
      n96 = local write "LBCB 2 Setting"(w118) -> ()
      n97 = call "ConsolidatedDAQChannelNames.vi"() -> ("Number of \nExternal \nChannels 1"=w120:i32)  [unwired: 5 out]
      n98 = local write "L1  Limits"(w97) -> ()
      n99 = call "Number Of LBCBs DAO.vi"("Actions"=w99) -> ("Number of\nLBCBs Out"=w101:T40)  [unwired: 3 in, 7 out]
      n100 = call "Auto Balance Error Tolerance DAO.vi"("Auto Balance Increment Actions"=w99, "LBCB Number"=w100) -> ("Auto Balance Error Out"=w116:T36)  [unwired: 3 in, 10 out]
      n101 = call "Auto Balance Error Tolerance DAO.vi"("Auto Balance Increment Actions"=w99, "LBCB Number"=w98) -> ("Auto Balance Error Out"=w117:T36)  [unwired: 3 in, 10 out]
      n102 = local write "Number of \nExternal \nChannels"(w120) -> ()
      n103 = call "Actuator Point 2 Array.vi"("Actuator Point"=w116) -> ("Array"=w114:dbl[])
      n104 = call "Actuator Point 2 Array.vi"("Actuator Point"=w117) -> ("Array"=w115:dbl[])
      n105 = local write "L1 Auto Balance Error Tolerance"(w114) -> ()
      n106 = local write "L2 Auto Balance Error Tolerance"(w115) -> ()
      n107 = call "Load Previous Command.vi"("Number of LBCBs"=w101) -> ()  [unwired: 3 out]
    }
  }
  n108 = call "External Sensor Sensitivities DAO.vi"("Persistent DAO Actions"=Persistant_DAO_Actions."Get") -> ("Sensitivities Out"=w16:dbl[])  [unwired: 3 in, 7 out]
  n109 = Obtain Notifier(name (unnamed)="Mixed Mode Statuses", notification data type=w60, error in (no error)=w13) -> (notifier out=w61:refnum<notifier>, error out=w15:errorcluster)  [unwired: 1 in, 1 out]
  n110 = Obtain Queue(name (unnamed)="Parameter Changes", element data type=T32 {"Change State"=enum."Mixed Mode", "LBCB Number"=enum."LBCB1"} ("Parameter Changes"), error in (no error)=w13) -> (queue out=w72:refnum<queue>, error out=w39:errorcluster)  [unwired: 2 in, 1 out]
  n111 = while {
    shift-right: [w193] -> _
    shift-left: _ -> [w190]
    shift-right: [w194] -> _
    shift-left: _ -> [w191]
    shift-right: [w195] -> _
    shift-left: _ -> [w192]
    tunnel: w16 -> [w189]
    shift-right: [w184] -> _
    shift-left: w61 -> [w185]
    tunnel: w60 -> [w183]
    tunnel: [w173] -> w48
    stop <- w173 stop-if-true
    w179 = T5 {"Displacements"=[], "Forces"=[]} ("LBCB 1 Measurements")
    w218 = 6 ("index")
    w198 = Actuator_Measurment_Actions."Set  Data" ("Measurement Actions")
    w227 = 6 ("index")
    w211 = T43 {"LVDTs"=[], " Commands"=[], "Load Cells"=[], "Servo"=[]} ("Actuator Data In")
    w210 = T44 {"Displacements"=[], "Forces"=[], "Displacement Commands"=[]} ("Cartesian Data In")
    # "Ramp time times a multiplier loosely aligned\nwith Nyquist's rule of thumb"
    # "Status Changes Loop"
    n112 = local read "MixedModeStates"() -> (w165:T24)
    n113 = local read "L2 Measurements"() -> (w206:T21)
    n114 = local read "External Sensors"() -> (w200:dbl[])
    n115 = local read "L1 Commands"() -> (w239:T10)
    n116 = local read "L2 Volts LVDT & LC"() -> (w212:dbl[])
    n117 = local read "L2 Commands"() -> (w207:T10)
    n118 = local read "L1 Measurements"() -> (w240:T21)
    n119 = local read "L1 Volts LVDT & LC"() -> (w228:dbl[])
    n120 = case shown="\"Init\", Default" w165 {
      tunnel: [FALSE TRUE TRUE TRUE TRUE TRUE TRUE TRUE TRUE TRUE TRUE TRUE] -> w158
      frame #0 {
      }
      frame #1 {
      }
      frame #2 {
      }
      frame #3 {
      }
      frame #4 {
      }
      frame #5 {
      }
      frame #6 {
      }
      frame #7 {
      }
      frame #8 {
      }
      frame #9 {
      }
      frame #10 {
      }
      frame #11 {
      }
    }
    n121 = Unbundle By Name(w207) -> ("Act Cmd"=w167:dbl[], "Cart Cmd"=w166:dbl[])
    n122 = Unbundle By Name(w206) -> ("Act Disp"=w205:dbl[], "Act Forces"=w204:dbl[], "Cart Disp"=w203:dbl[], "Cart Forces"=w202:dbl[])
    n123 = Unbundle By Name(w240) -> ("Act Disp"=w238:dbl[], "Act Forces"=w237:dbl[], "Cart Disp"=w236:dbl[], "Cart Forces"=w235:dbl[])
    n124 = local read "L1 Servo Error"() -> (w224:dbl[])
    n125 = Unbundle By Name(w239) -> ("Act Cmd"=w169:dbl[], "Cart Cmd"=w168:dbl[])
    n126 = local read "Averaging"() -> (w199:bool)
    n127 = Multiply(x=w200, y=w189) -> (x*y=w201:dbl[])
    n128 = local read "L2 Servo Error"() -> (w208:dbl[])
    n129 = local read "L2 Cmd  Volts"() -> (w209:dbl[])
    n130 = Delete From Array(array=w212, length=w218, index=w218) -> (deleted portion=w219:dbl[], array with subset deleted=w220:dbl[])
    n131 = local read "L1 Cmd  Volts"() -> (w229:dbl[])
    n132 = Delete From Array(array=w228, length=w227, index=w227) -> (deleted portion=w226:dbl[], array with subset deleted=w225:dbl[])
    n133 = call "Sample Averaging.vi"("Sample In"=w205, "Averaging"=w199) -> ("Sample Out"=w215:dbl[])  [unwired: 9 out]
    n134 = call "Sample Averaging.vi"("Sample In"=w204, "Averaging"=w199) -> ("Sample Out"=w216:dbl[])  [unwired: 9 out]
    n135 = call "Sample Averaging.vi"("Sample In"=w203, "Averaging"=w199) -> ("Sample Out"=w217:dbl[])  [unwired: 9 out]
    n136 = call "Sample Averaging.vi"("Sample In"=w202, "Averaging"=w199) -> ("Sample Out"=w175:dbl[])  [unwired: 9 out]
    n137 = call "Sample Averaging.vi"("Sample In"=w201, "Averaging"=w199) -> ("Sample Out"=w157:dbl[])  [unwired: 9 out]
    n138 = call "Sample Averaging.vi"("Sample In"=w238, "Averaging"=w199) -> ("Sample Out"=w232:dbl[])  [unwired: 9 out]
    n139 = call "Sample Averaging.vi"("Sample In"=w237, "Averaging"=w199) -> ("Sample Out"=w231:dbl[])  [unwired: 9 out]
    n140 = call "Sample Averaging.vi"("Sample In"=w236, "Averaging"=w199) -> ("Sample Out"=w230:dbl[])  [unwired: 9 out]
    n141 = call "Sample Averaging.vi"("Sample In"=w235, "Averaging"=w199) -> ("Sample Out"=w176:dbl[])  [unwired: 9 out]
    n142 = local read "L2 Current Target"() -> (w163:T6)
    n143 = local read "L1 Current Target"() -> (w164:T6)
    n144 = local read "L2 Iterative Target"() -> (w159:T6)
    n145 = local read "L1 Iterative Target"() -> (w160:T6)
    n146 = local read "L1 Convergence Status"() -> (w181:T23)
    n147 = local read "L2 Convergence Status"() -> (w180:T23)
    n148 = Bundle By Name(cluster=w210, "Displacements"=w230, "Forces"=w176, "Displacement Commands"=w168) -> (w223:T44)
    n149 = Bundle By Name(cluster=w210, "Displacements"=w217, "Forces"=w175, "Displacement Commands"=w166) -> (w221:T44)
    n150 = Bundle By Name(cluster=w211, "LVDTs"=w215, "Commands"=w167, "Load Cells"=w216) -> (w213:T43)
    n151 = Bundle By Name(cluster=w211, "LVDTs"=w220, "Commands"=w209, "Load Cells"=w219, "Servo"=w208) -> (w214:T43)
    n152 = Bundle By Name(cluster=w211, "LVDTs"=w232, "Commands"=w169, "Load Cells"=w231) -> (w234:T43)
    n153 = Bundle By Name(cluster=w211, "LVDTs"=w225, "Commands"=w229, "Load Cells"=w226, "Servo"=w224) -> (w233:T43)
    n154 = Select(t=w160, s=w158, f=w164) -> (s? t:f=w162:T6)
    n155 = call "Actuator Data Set.vi"("Selected LBCB"=LBCB_Number."LBCB2", "Volts In"=w214, "Actuator Data In"=w213, "Measurement Actions"=w198) -> ()  [unwired: 1 in, 7 out]
    n156 = Select(t=w159, s=w158, f=w163) -> (s? t:f=w161:T6)
    n157 = call "Actuator Data Set.vi"("Selected LBCB"=LBCB_Number."LBCB1", "Volts In"=w233, "Actuator Data In"=w234, "Measurement Actions"=w198) -> ()  [unwired: 1 in, 7 out]
    n158 = call "GetSamplingRate.vi"() -> ("Sampling"=w174:i32)
    n159 = local read "App Running"() -> (w241:bool)
    n160 = Bundle By Name(cluster=w179, "Displacements"=w168, "Forces"=w176) -> (w178:T5)
    n161 = Bundle By Name(cluster=w179, "Displacements"=w166, "Forces"=w175) -> (w177:T5)
    n162 = local read "Ramp Time"() -> (w188:u32)
    n163 = local read "L1 Autobalance Out"() -> (w172:T1[])
    n164 = local read "L2 Autobalance Out"() -> (w171:T1[])
    n165 = local read "Hold Period"() -> (w196:bool)
    n166 = Not(x=w241) -> (.not. x?=w173:bool)
    n167 = local write "Status Changes"(w174) -> ()
    n168 = Bundle By Name(cluster=w183, "LBCB  1 Target"=w162, "LBCB 2 Target"=w161, "MixedModeStates"=w165, "LBCB 1 Convergence"=w181, "LBCB 2 Convergence"=w180, "LBCB 1 Measurements"=w178, "LBCB 2 Measurements"=w177) -> (w182:T30)
    n169 = case shown="True" w196 {
      tunnel: w157 -> [w257 w266]
      tunnel: w223 -> [w258 w267]
      tunnel: w221 -> [w256 w265]
      tunnel: [w258 w261] -> w195
      tunnel: [w257 w262] -> w194
      tunnel: [w256 w260] -> w193
      tunnel: w192 -> [_ w261]
      tunnel: w191 -> [_ w262]
      tunnel: w190 -> [_ w260]
      frame #0 {
        w259 = Cartesian_Measurment_Actions."Set Data" ("Measurement Actions")
        n170 = call "Cartesian Data Set.vi"("Measurement Actions"=w259, "Cartesian Data In"=w256, "LBCB Selected"=LBCB_Number."LBCB2", "Cartesian Hold Data In"=w256) -> ()  [unwired: 2 in, 10 out]
        n171 = call "External Sensors Data Set.vi"("Hold  Data In"=w257, "Input Data"=w257, "Measurement Actions"=w259) -> ()  [unwired: 1 in, 8 out]
        n172 = call "Cartesian Data Set.vi"("Measurement Actions"=w259, "Cartesian Data In"=w258, "LBCB Selected"=LBCB_Number."LBCB1", "Cartesian Hold Data In"=w258) -> ()  [unwired: 2 in, 10 out]
      }
      frame #1 {
        w268 = Cartesian_Measurment_Actions."Set Data" ("Measurement Actions")
        n173 = call "Cartesian Data Set.vi"("Measurement Actions"=w268, "Cartesian Data In"=w265, "LBCB Selected"=LBCB_Number."LBCB2", "Cartesian Hold Data In"=w260) -> ()  [unwired: 2 in, 10 out]
        n174 = call "External Sensors Data Set.vi"("Hold  Data In"=w266, "Input Data"=w266, "Measurement Actions"=w268) -> ()  [unwired: 1 in, 8 out]
        n175 = call "Cartesian Data Set.vi"("Measurement Actions"=w268, "Cartesian Data In"=w267, "LBCB Selected"=LBCB_Number."LBCB1", "Cartesian Hold Data In"=w261) -> ()  [unwired: 2 in, 10 out]
      }
    }
    n176 = Multiply(x=w188, y=u32 2) -> (x*y=w186:u32)
    n177 = Wait Until Next ms Multiple(millisecond multiple=w186) -> ()  [unwired: 1 out]
    n178 = call "Autobalance Data DAO.vi"("L2 Autobalance In"=w171, "L1 Autobalance Iin"=w172, "DAO Actions"=DAO_Actions."Set") -> ()  [unwired: 1 in, 8 out]
    n179 = Send Notification(notification=w182, notifier=w185) -> (notifier out=w184:refnum<notifier>)  [unwired: 1 in, 1 out]
  }
  n180 = Flush Queue(queue=w72, error in (no error)=w39) -> (queue out=w40:refnum<queue>, error out=w38:errorcluster)  [unwired: 1 out]
  n181 = call "Number Of LBCBs DAO.vi"("Actions"=Persistant_DAO_Actions."Get") -> ("Number of\nLBCBs Out"=w4:T40)  [unwired: 3 in, 7 out]
  n182 = flat-sequence {
    tunnel: [w275] -> w21
    tunnel: [w277] -> w20
    tunnel: [w276] -> w19
    tunnel: w13 -> [_]
    tunnel: [w270] -> w10
    tunnel: [w269] -> w6
    frame #0 {
      n183 = global read "Global Cache.vi" "L2 Calibrations"() -> (w278:T46)
      n184 = global read "Global Cache.vi" "Autobalance \nControl Parameters"() -> (w269:T47)
      n185 = Unbundle By Name(w278) -> ("Command Sensitivity"=w275:dbl[], "Servo Error Offset"=w270:dbl[], "LVDT Sensitivity"=w272:dbl[], "LVDT Offset"=w274:dbl[], "Load Cell Offsets"=w273:dbl[], "Load Cell Sensitivity"=w271:dbl[])
      n186 = Build Array (concatenate)(w274, w273) -> (w277:dbl[])
      n187 = Build Array (concatenate)(w272, w271) -> (w276:dbl[])
    }
  }
  n188 = call "Init Mixed Mode Command.vi"("error in (no error)"=w15) -> ("Command Data"=w35:T6)  [unwired: 2 out]
  n189 = Obtain Queue(name (unnamed)="Mixed Mode Commands", element data type=w3, error in (no error)=w15) -> (queue out=w71:refnum<queue>, error out=w68:errorcluster)  [unwired: 2 in, 1 out]
  n190 = Bundle By Name(cluster=w3, "Command"=Mixed_Mode_Command_Action."No Op", "Ramp Times"=cluster{"Initial":T27, "Iterative":T27} {"Initial"={"Ramp"=0.0, "Stab"=0.0, "Hold"=0.0}, "Iterative"={"Ramp"=0.0, "Stab"=0.0, "Hold"=0.0}}, "LBCB1"=w35, "LBCB2"=w35) -> (w34:T31)
  n191 = Flush Queue(queue=w71, error in (no error)=w68) -> (queue out=w2:refnum<queue>, error out=w14:errorcluster)  [unwired: 1 out]
  n192 = while {
    shift-right: [w290] -> _
    shift-left: w40 -> [w293]
    shift-right: [w282] -> _
    shift-left: w38 -> [w292]
    tunnel: [w286] -> w49
    tunnel: w9 -> [w285]
    tunnel: w4 -> [w284]
    tunnel: w3 -> [w281]
    shift-right: [w279] -> _
    shift-left: w2 -> [w280]
    stop <- w286 stop-if-true
    # "Parameter Changes Loop"
    n193 = Dequeue Element(queue=w293, timeout in ms (-1)=2000, error in (no error)=w292) -> (queue out=w290:refnum<queue>, element=w289:T32, timed out?=w291:bool, error out=w283:errorcluster)
    n194 = case shown="False" w291 {
      tunnel: w289 -> [w303 _]
      tunnel: w285 -> [w300 _]
      tunnel: w284 -> [w299 _]
      tunnel: w283 -> [w298 w449]
      tunnel: [w297 w449] -> w282
      tunnel: w281 -> [w296 _]
      tunnel: w280 -> [w295 w450]
      tunnel: [w294 w450] -> w279
      frame #0 {
        n195 = Unbundle By Name(w303) -> ("Change State"=w302:T33, "LBCB Number"=w301:T29)
        n196 = case shown="\"Stop Application\"" w302 {
          tunnel: w301 -> [_ _ _ _ _ w390 _ w399 w409 w442 _]
          tunnel: w300 -> [_ _ _ w372 _ _ _ _ _ _ _]
          tunnel: w299 -> [_ _ _ _ _ _ _ _ w410 _ _]
          tunnel: w298 -> [w305 w324 w332 w351 w379 w389 w395 w398 w407 w441 w447]
          tunnel: [w305 w324 w332 w351 w379 w389 w395 w398 w406 w441 w447] -> w297
          tunnel: w296 -> [_ _ _ _ _ _ _ _ w405 _ _]
          tunnel: w295 -> [w304 w323 w331 w350 w378 w388 w394 w397 w404 w440 w446]
          tunnel: [w304 w323 w331 w350 w378 w388 w394 w397 w403 w440 w446] -> w294
          frame #0 {
            w318 = LBCB_Number."LBCB2" ("LBCB Number")
            w319 = LBCB_Number."LBCB1" ("LBCB Number")
            w320 = Persistant_DAO_Actions."Get" ("LBCB Settings Actions")
            n197 = call "Mixed Mode Force Error Range DAO.vi"("Force Error Range Actions"=w320, "LBCB Number"=w319) -> ("Force Error Range Out"=w317:T34)  [unwired: 3 in, 10 out]
            n198 = call "Mixed Mode Jacobian Gain DAO.vi"("Jacobian Gain Actions"=w320, "LBCB Number"=w319) -> ("Jacobian Gain Out"=w316:T34)  [unwired: 3 in, 10 out]
            n199 = call "Mixed Mode Max Increment DAO.vi"("Max Increment Actions"=w320, "LBCB Number"=w319) -> ("Max Increment Out"=w315:T34)  [unwired: 3 in, 10 out]
            n200 = call "LBCB Position DAO.vi"("LBCB Settings Actions"=w320, "LBCB Number"=w319) -> ("LBCB Position Output"=w322:T20)  [unwired: 3 in, 10 out]
            n201 = call "LBCB Position DAO.vi"("LBCB Settings Actions"=w320, "LBCB Number"=w318) -> ("LBCB Position Output"=w321:T20)  [unwired: 3 in, 10 out]
            n202 = call "Cartesian Point 2 Array.vi"("Cart Disp"=w317) -> ("Array"=w314:dbl[])  [unwired: 2 out]
            n203 = call "Cartesian Point 2 Array.vi"("Cart Disp"=w316) -> ("Array"=w313:dbl[])  [unwired: 2 out]
            n204 = call "Cartesian Point 2 Array.vi"("Cart Disp"=w315) -> ("Array"=w312:dbl[])  [unwired: 2 out]
            n205 = call "Mixed Mode Force Error Range DAO.vi"("Force Error Range Actions"=w320, "LBCB Number"=w318) -> ("Force Error Range Out"=w308:T34)  [unwired: 3 in, 10 out]
            n206 = call "Mixed Mode Jacobian Gain DAO.vi"("Jacobian Gain Actions"=w320, "LBCB Number"=w318) -> ("Jacobian Gain Out"=w307:T34)  [unwired: 3 in, 10 out]
            n207 = local write "L1  Position"(w322) -> ()
            n208 = local write "L2 Position"(w321) -> ()
            n209 = call "Cartesian Point 2 Array.vi"("Cart Disp"=w308) -> ("Array"=w311:dbl[])  [unwired: 1 in, 1 out]
            n210 = call "Cartesian Point 2 Array.vi"("Cart Disp"=w307) -> ("Array"=w310:dbl[])  [unwired: 1 in, 1 out]
            n211 = call "Mixed Mode Max Increment DAO.vi"("Max Increment Actions"=w320, "LBCB Number"=w318) -> ("Max Increment Out"=w306:T34)  [unwired: 3 in, 10 out]
            n212 = local write "L1 Max Increment"(w312) -> ()
            n213 = local write "L1 Jacobian Gain"(w313) -> ()
            n214 = local write "L1 Force Error Range"(w314) -> ()
            n215 = call "Cartesian Point 2 Array.vi"("Cart Disp"=w306) -> ("Array"=w309:dbl[])  [unwired: 1 in, 1 out]
            n216 = local write "L2 Jacobian Gain"(w310) -> ()
            n217 = local write "L2 Force Error Range"(w311) -> ()
            n218 = local write "L2 Max Increment"(w309) -> ()
          }
          frame #1 {
            w326 = Persistant_DAO_Actions."Set" ("Actions")
            w329 = LBCB_Number."LBCB1" ("LBCB Number")
            w328 = LBCB_Number."LBCB2" ("LBCB Number")
            w330 = Persistant_DAO_Actions."Get" ("Actions")
            n219 = call "Stiffness Jacobian DAO.vi"("LBCB Number"=w329, "Actions"=w330) -> ("Stiffness Jacobian Out"=w327:T22)  [unwired: 3 in, 6 out]
            n220 = call "Stiffness Jacobian DAO.vi"("LBCB Number"=w328, "Actions"=w330) -> ("Stiffness Jacobian Out"=w325:T22)  [unwired: 3 in, 6 out]
            n221 = call "Calculated Stiffness Jacobian.vi"("Stiffness Jacobian In"=w327, "LBCB Number"=w329, "Actions"=w326) -> ()  [unwired: 1 in, 8 out]
            n222 = call "Calculated Stiffness Jacobian.vi"("Stiffness Jacobian In"=w325, "LBCB Number"=w328, "Actions"=w326) -> ()  [unwired: 1 in, 8 out]
            n223 = local write "L1 Stiffness Jacobian"(w327) -> ()
            n224 = local write "L2 Stiffness Jacobian"(w325) -> ()
          }
          frame #2 {
            w334 = LBCB_Number."LBCB2" ("LBCB Number")
            w335 = LBCB_Number."LBCB1" ("LBCB Number")
            w333 = Persistant_DAO_Actions."Get" ("I Gain Actions")
            n225 = call "I Gain DAO.vi"("I Gain Actions"=w333, "LBCB Number"=w335) -> ("I Gain"=w349:T36)  [unwired: 3 in, 10 out]
            n226 = call "P Gain DAO.vi"("P Gain Actions"=w333, "LBCB Number"=w335) -> ("P Gain"=w348:T36)  [unwired: 3 in, 10 out]
            n227 = call "PID Controls DAO.vi"("Actions"=w333) -> ("PID Control  Out"=w345:T8)  [unwired: 3 in, 7 out]
            n228 = call "I Gain DAO.vi"("I Gain Actions"=w333, "LBCB Number"=w334) -> ("I Gain"=w343:T36)  [unwired: 3 in, 10 out]
            n229 = call "P Gain DAO.vi"("P Gain Actions"=w333, "LBCB Number"=w334) -> ("P Gain"=w344:T36)  [unwired: 3 in, 10 out]
            n230 = call "PID Controls DAO.vi"("Actions"=w333) -> ("PID Control  Out"=w342:T8)  [unwired: 3 in, 7 out]
            n231 = local write "L2 PID Control"(w342) -> ()
            n232 = call "Actuator Point 2 Array.vi"("Actuator Point"=w349) -> ("Array"=w347:dbl[])
            n233 = call "Actuator Point 2 Array.vi"("Actuator Point"=w348) -> ("Array"=w346:dbl[])
            n234 = call "Actuator Point 2 Array.vi"("Actuator Point"=w343) -> ("Array"=w341:dbl[])
            n235 = call "Actuator Point 2 Array.vi"("Actuator Point"=w344) -> ("Array"=w340:dbl[])
            n236 = local write "L2 P Gain"(w340) -> ()
            n237 = local write "L2 I Gain"(w341) -> ()
            n238 = local write "L1 P Gain"(w346) -> ()
            n239 = local write "L1 I Gain"(w347) -> ()
            n240 = local write "L1 PID Control"(w345) -> ()
            n241 = call "Auto Balance Error Tolerance DAO.vi"("Auto Balance Increment Actions"=w333, "LBCB Number"=w335) -> ("Auto Balance Error Out"=w339:T36)  [unwired: 3 in, 10 out]
            n242 = call "Auto Balance Error Tolerance DAO.vi"("Auto Balance Increment Actions"=w333, "LBCB Number"=w334) -> ("Auto Balance Error Out"=w338:T36)  [unwired: 3 in, 10 out]
            n243 = call "Actuator Point 2 Array.vi"("Actuator Point"=w339) -> ("Array"=w336:dbl[])
            n244 = call "Actuator Point 2 Array.vi"("Actuator Point"=w338) -> ("Array"=w337:dbl[])
            n245 = local write "L2 Auto Balance Error Tolerance"(w337) -> ()
            n246 = local write "L1 Auto Balance Error Tolerance"(w336) -> ()
          }
          frame #3 {
            w375 = LBCB_Number."LBCB2" ("ID")
            w376 = LBCB_Number."LBCB1" ("ID")
            w377 = Persistant_DAO_Actions."Get" ("Actuator Force Limit Actions")
            n247 = call "Actuator Force Limit DAO.vi"("Actuator Force Limit Actions"=w377, "ID"=w376) -> ("Actuator Force Limits Out"=w371:T35)  [unwired: 3 in, 10 out]
            n248 = call "Actuator Stroke Limit DAO.vi"("Actuator Stroke Limit Actions"=w377, "ID"=w376) -> ("Actuator Stroke Limits Out"=w370:T35)  [unwired: 3 in, 10 out]
            n249 = call "Cartesian Displacement Limit DAO.vi"("Cartesian Displacement Limit Actions"=w377, "ID"=w376) -> ("Cartesian Displacement Out"=w369:T37)  [unwired: 3 in, 10 out]
            n250 = call "Cartesian Force Limit DAO.vi"("Cartesian Force Limit Actions"=w377, "ID"=w376) -> ("Cartesian Force Limit Out"=w368:T37)  [unwired: 3 in, 10 out]
            n251 = call "Command Voltage Limit DAO.vi"("Actuator Stroke Limit Actions"=w377, "ID"=w376) -> ("Command Voltage Limit Out"=w367:T35)  [unwired: 3 in, 10 out]
            n252 = call "Cartesian Matrix 2 2D Array.vi"("Matrix In"=w369) -> ("Matrix Out"=w364:T19)  [unwired: 10 out]
            n253 = call "Actuator Matrix 2 2D Array.vi"("Matrix In"=w371) -> ("Matrix Out"=w366:T19)  [unwired: 10 out]
            n254 = call "Actuator Matrix 2 2D Array.vi"("Matrix In"=w370) -> ("Matrix Out"=w365:T19)  [unwired: 10 out]
            n255 = call "Cartesian Matrix 2 2D Array.vi"("Matrix In"=w368) -> ("Matrix Out"=w363:T19)  [unwired: 10 out]
            n256 = call "Actuator Matrix 2 2D Array.vi"("Matrix In"=w367) -> ("Matrix Out"=w362:T19)  [unwired: 10 out]
            n257 = Bundle By Name(cluster=w372, "Actuator Force Limits"=w366, "Actuator Stroke Limits"=w365, "Cartesian Disp Limit"=w364, "Cartesian Force Limit"=w363, "Command Voltage Limit"=w362) -> (w374:T18)
            n258 = call "Actuator Force Limit DAO.vi"("Actuator Force Limit Actions"=w377, "ID"=w375) -> ("Actuator Force Limits Out"=w361:T35)  [unwired: 3 in, 10 out]
            n259 = call "Actuator Stroke Limit DAO.vi"("Actuator Stroke Limit Actions"=w377, "ID"=w375) -> ("Actuator Stroke Limits Out"=w360:T35)  [unwired: 3 in, 10 out]
            n260 = call "Cartesian Displacement Limit DAO.vi"("Cartesian Displacement Limit Actions"=w377, "ID"=w375) -> ("Cartesian Displacement Out"=w359:T37)  [unwired: 3 in, 10 out]
            n261 = call "Cartesian Force Limit DAO.vi"("Cartesian Force Limit Actions"=w377, "ID"=w375) -> ("Cartesian Force Limit Out"=w358:T37)  [unwired: 3 in, 10 out]
            n262 = call "Command Voltage Limit DAO.vi"("Actuator Stroke Limit Actions"=w377, "ID"=w375) -> ("Command Voltage Limit Out"=w357:T35)  [unwired: 3 in, 10 out]
            n263 = call "Cartesian Matrix 2 2D Array.vi"("Matrix In"=w358) -> ("Matrix Out"=w353:T19)  [unwired: 10 out]
            n264 = call "Cartesian Matrix 2 2D Array.vi"("Matrix In"=w359) -> ("Matrix Out"=w354:T19)  [unwired: 10 out]
            n265 = call "Actuator Matrix 2 2D Array.vi"("Matrix In"=w361) -> ("Matrix Out"=w356:T19)  [unwired: 10 out]
            n266 = call "Actuator Matrix 2 2D Array.vi"("Matrix In"=w360) -> ("Matrix Out"=w355:T19)  [unwired: 10 out]
            n267 = call "Actuator Matrix 2 2D Array.vi"("Matrix In"=w357) -> ("Matrix Out"=w352:T19)  [unwired: 10 out]
            n268 = Bundle By Name(cluster=w372, "Actuator Force Limits"=w356, "Actuator Stroke Limits"=w355, "Cartesian Disp Limit"=w354, "Cartesian Force Limit"=w353, "Command Voltage Limit"=w352) -> (w373:T18)
            n269 = local write "L1  Limits"(w374) -> ()
            n270 = local write "L2 Limits"(w373) -> ()
          }
          frame #4 {
            w380 = 1000.0 ("x")
            n271 = call "App Parameters DAO.vi"("Actions"=Persistant_DAO_Actions."Get") -> ("Application Timing and Logging Out"=w386:T38)  [unwired: 3 in, 7 out]
            n272 = Unbundle By Name(w386) -> ("Ramp Time.Interval"=w385:dbl, "Logging Directory"=w383:path, "Volt Logging Loop.Interval"=w382:dbl)
            n273 = Multiply(x=w380, y=w382) -> (x*y=w381:dbl)
            n274 = Multiply(x=w380, y=w385) -> (x*y=w384:dbl)
            n275 = local write "Volt Logger Time"(w381) -> ()
            n276 = local write "Logging Directory"(w383) -> ()
            n277 = local write "Ramp Time"(w384) -> ()
          }
          frame #5 {
            n278 = case shown="\"LBCB1\"" w390 {
              tunnel: Control_Loop_State."Reset Autobalancing" ("L1 Ctrl Loop State") -> [w392 w393]
              frame #0 {
                n279 = local write "L1 Ctrl Loop State"(w392) -> ()
              }
              frame #1 {
                n280 = local write "L2 Ctrl Loop State"(w393) -> ()
              }
            }
          }
          frame #6 {
            n281 = local write "App Running"(FALSE ("App Running")) -> ()
          }
          frame #7 {
            n282 = case shown="\"LBCB1\"" w399 {
              tunnel: Control_Loop_State."Set Command" ("L1 Ctrl Loop State") -> [w401 w402]
              frame #0 {
                n283 = local write "L1 Ctrl Loop State"(w401) -> ()
              }
              frame #1 {
                n284 = local write "L2 Ctrl Loop State"(w402) -> ()
              }
            }
          }
          frame #8 {
            w408 = Control_Loop_State."On" ("L1 Ctrl Loop State")
            n285 = case shown="\"2\"" w410 {
              tunnel: w409 -> [_ w420]
              tunnel: w408 -> [_ w419]
              tunnel: w407 -> [w412 w417]
              tunnel: [w412 w416] -> w406
              tunnel: w405 -> [_ w415]
              tunnel: w404 -> [w411 w414]
              tunnel: [w411 w413] -> w403
              frame #0 {
              }
              frame #1 {
                n286 = case shown="\"LBCB2\"" w420 {
                  tunnel: w419 -> [w433 w436]
                  tunnel: [w432 w435] -> w418
                  frame #0 {
                    n287 = local read "L2 Ctrl Loop State"() -> (w434:T9)
                    n288 = Equal?(x=w433, y=w434) -> (x = y?=w432:bool)
                  }
                  frame #1 {
                    n289 = local read "L1 Ctrl Loop State"() -> (w437:T9)
                    n290 = Equal?(x=w436, y=w437) -> (x = y?=w435:bool)
                  }
                }
                n291 = case shown="True" w418 {
                  tunnel: w417 -> [w422 w431]
                  tunnel: [w422 w430] -> w416
                  tunnel: w415 -> [_ w428]
                  tunnel: w414 -> [w421 w427]
                  tunnel: [w421 w426] -> w413
                  frame #0 {
                  }
                  frame #1 {
                    n292 = call "Default Ramp Time DAO.vi"("Ramp Time Actions"=Persistant_DAO_Actions."Get") -> ("Ramp Time Out"=w423:T49)  [unwired: 12 in, 2 out]
                    n293 = Bundle By Name(cluster=w428, "Command"=Mixed_Mode_Command_Action."Measure Initial Position", "Ramp Times"=w423) -> (w429:T31)
                    n294 = Enqueue Element(queue=w427, element=w429, error in (no error)=w431) -> (queue out=w426:refnum<queue>, error out=w430:errorcluster)  [unwired: 1 in, 1 out]
                  }
                }
              }
            }
            n295 = case shown="\"LBCB1\"" w409 {
              tunnel: w408 -> [w438 w439]
              frame #0 {
                n296 = local write "L1 Ctrl Loop State"(w438) -> ()
              }
              frame #1 {
                n297 = local write "L2 Ctrl Loop State"(w439) -> ()
              }
            }
          }
          frame #9 {
            n298 = case shown="\"LBCB1\"" w442 {
              tunnel: Control_Loop_State."Ready for Control" ("L1 Ctrl Loop State") -> [w444 w445]
              frame #0 {
                n299 = local write "L1 Ctrl Loop State"(w444) -> ()
              }
              frame #1 {
                n300 = local write "L2 Ctrl Loop State"(w445) -> ()
              }
            }
          }
          frame #10 {
            n301 = local write "DAQ Enabled"(TRUE ("DAQ Enabled")) -> ()
          }
        }
      }
      frame #1 {
        n302 = local read "L1 Ctrl Loop State"() -> (w456:T9)
        n303 = local read "L2 Ctrl Loop State"() -> (w453:T9)
        n304 = call "App Status Globals.vi"("App Status Actions"=App_Status_Actions."Get Status") -> ("App Status Out"=w460:T51)  [unwired: 5 in, 9 out]
        n305 = call "Control Loop State 2 Flags.vi"("L1 Ctrl Loop State"=w456) -> ("Controlled"=w454:bool, "Autobalanced"=w455:bool)
        n306 = local read "DAQ Started"() -> (w457:bool)
        n307 = call "Control Loop State 2 Flags.vi"("L1 Ctrl Loop State"=w453) -> ("Controlled"=w452:bool, "Autobalanced"=w451:bool)
        n308 = Bundle By Name(cluster=w460, "Controlling L2"=w452, "Autobalance L2"=w451, "Data Acquisition"=w457, "Controlling L1"=w454, "Autobalance L1"=w455) -> (w458:T51)
        n309 = call "App Status Globals.vi"("App Status Actions"=App_Status_Actions."Set All", "App Status In"=w458) -> ()  [unwired: 4 in, 10 out]
      }
    }
    n310 = local read "App Running"() -> (w288:bool)
    n311 = Not(x=w288) -> (.not. x?=w286:bool)
  }
  n312 = Obtain Notifier(name (unnamed)="Mixed Mode State", notification data type=w70, error in (no error)=w14) -> (notifier out=w53:refnum<notifier>, error out=w67:errorcluster)  [unwired: 1 in, 1 out]
  n313 = while {
    shift-right: [w487] -> _
    shift-left: w70 -> [w503]
    shift-right: [w513] -> _
    shift-left: _ -> [w508]
    shift-right: [w511] -> _
    shift-left: u32 0 ("New Start Time") -> [w509]
    shift-right: [w506] -> _
    shift-left: w53 -> [w507]
    shift-right: [w498] -> _
    shift-left: w67 -> [w505]
    shift-right: [w477] -> _
    shift-left: w66 -> [w490]
    shift-right: [w488] -> _
    shift-left: w66 -> [w489]
    shift-right: [w502] -> _
    shift-left: w70 -> [w501]
    shift-right: [w499] -> _
    shift-left: w2 -> [w500]
    shift-right: [w493] -> _
    shift-left: w34 -> [w497]
    tunnel: [w480] -> w47
    shift-right: [w478] -> _
    shift-left: FALSE ("DAQ Started") -> [w479]
    tunnel: w4 -> [w475]
    tunnel: w4 -> [w462]
    stop <- w480 stop-if-true
    # "Send Cmd"
    # "Prev\nReading"
    # "Collect"
    # "PID Hold"
    # "Hold"
    # "Average"
    n314 = Unbundle By Name(w497) -> ("Command"=w496:T28)
    n315 = case shown="\"Exit\"" w496 {
      tunnel: w503 -> [w1176 _ _ w1179 w1180 w1181]
      tunnel: [w1176 Mixed_Mode_States."Aborting" ("MixedModeStates") Mixed_Mode_States."Exit" ("MixedModeStates") w1179 w1180 w1181] -> w514
      frame #0 {
      }
      frame #1 {
      }
      frame #2 {
      }
      frame #3 {
      }
      frame #4 {
      }
      frame #5 {
      }
    }
    n316 = call "GetSamplingRate.vi"() -> ("Sampling"=w481:i32)
    n317 = local write "Mixed Mode"(w481) -> ()
    n318 = call "Ramp Timer.vi"("Previous Ramp Time"=w509) -> ("New Start Time"=w510:u32, "Current Ramp Time"=w512:u64)
    n319 = local read "L1  Position"() -> (w465:T20)
    n320 = local read "LBCB 1 Setting"() -> (w467:T15)
    n321 = local read "L2 Position"() -> (w463:T20)
    n322 = local read "LBCB 2 Setting"() -> (w468:T15)
    n323 = local read "Ramp Time"() -> (w476:u32)
    n324 = Unbundle By Name(w467) -> ("Type"=w466:T17)
    n325 = Unbundle By Name(w468) -> ("Type"=w464:T17)
    n326 = local read "L2 Commands"() -> (w474:T10)
    n327 = local read "L1 Ctrl Loop Out Actuator"() -> (w470:dbl[])
    n328 = local read "L1 Commands"() -> (w471:T10)
    n329 = local read "L2 Ctrl Loop Out Actuator"() -> (w473:dbl[])
    n330 = Bundle By Name(cluster=w471, "Act Cmd"=w470) -> (w469:T10)
    n331 = Bundle By Name(cluster=w474, "Act Cmd"=w473) -> (w472:T10)
    n332 = case shown="\"Start Initial Ramp\"" w514 {
      selector: w514 -> [w525 w566 w588 w601 w614 w659 w711 w736 w772 w813 w865 w901 w934 w956 w970 w984 w998 w1012 w1026 w1040 w1054 w1068 w1078 w1086 w1093]
      tunnel: [Mixed_Mode_States."Wait For DAQ" ("f") w569 w592 Mixed_Mode_States."Initial Position" ("MixedModeStates") w623 w662 w701 Mixed_Mode_States."Convergence Check" ("MixedModeStates") w789 Mixed_Mode_States."Update Command" ("MixedModeStates") Mixed_Mode_States."Start Iterative Ramp" ("MixedModeStates") Mixed_Mode_States."Run Iterative Ramp" ("MixedModeStates") w933 Mixed_Mode_States."Iterative Stabilize" ("MixedModeStates") w977 Mixed_Mode_States."Iterative Holding" ("MixedModeStates") w1007 Mixed_Mode_States."Stabilize" ("MixedModeStates") w1033 Mixed_Mode_States."Holding" ("MixedModeStates") w1063 Mixed_Mode_States."Idle" ("f") Mixed_Mode_States."Done" ("f") Mixed_Mode_States."Exit" ("f") Mixed_Mode_States."Idle" ("f")] -> w487
      tunnel: [T27 {"Ramp"=0.0, "Stab"=0.0, "Hold"=0.0} ("Initial") w572 w596 w597 w620 w645 w712 w751 w788 w823 w874 w906 w935 w957 w971 w987 w1004 w1013 w1027 w1043 w1060 w1072 w1082 w1087 w1096] -> w513
      tunnel: w512 -> [_ _ _ _ w617 _ w714 _ _ _ _ _ w937 _ w973 _ w1001 _ w1029 _ w1057 _ _ _ _]
      tunnel: [w528 w571 w595 w602 w624 w661 w713 w742 w787 w822 w872 w908 w936 w958 w980 w985 w1008 w1014 w1036 w1041 w1064 w1071 w1080 w1089 w1094] -> w511
      tunnel: w510 -> [_ _ _ w602 _ w661 _ _ _ _ _ w908 _ w958 _ w985 _ w1014 _ w1041 _ _ _ _ _]
      tunnel: w509 -> [w528 w571 w595 _ w624 _ w713 w742 w787 w822 w872 _ w936 _ w980 _ w1008 _ w1036 _ w1064 w1071 w1080 w1089 w1094]
      tunnel: w508 -> [_ w572 w596 _ w620 _ w712 w751 w788 w823 w874 _ w935 _ w971 w987 w1004 _ w1027 w1043 w1060 w1072 w1082 w1087 w1096]
      tunnel: w496 -> [_ w536 w593 _ _ _ _ _ _ _ _ _ _ _ _ _ _ _ _ _ _ _ _ _ _]
      tunnel: w490 -> [_ _ _ _ _ _ _ _ _ w807 _ _ _ _ _ _ _ _ _ _ _ _ _ _ _]
      tunnel: w489 -> [_ _ _ _ _ _ _ _ _ w808 _ _ _ _ _ _ _ _ _ _ _ _ _ _ _]
      tunnel: [w525 w566 w588 w601 w614 w659 w711 w736 w772 w813 w865 w901 w934 w956 w970 w984 w998 w1012 w1026 w1040 w1054 w1068 w1078 w1086 w1093] -> w502
      tunnel: w501 -> [_ _ _ _ _ _ _ _ w774 _ _ _ _ _ _ _ _ _ _ _ _ _ _ _ _]
      tunnel: w500 -> [w524 w565 w587 w600 w611 w649 w696 w735 w763 w811 w864 w900 w917 w955 w967 w982 w994 w1011 w1023 w1039 w1051 w1066 w1076 w1084 w1092]
      tunnel: [w524 w564 w586 w600 w610 w649 w695 w735 w763 w811 w864 w900 w916 w955 w966 w982 w993 w1011 w1022 w1039 w1050 w1066 w1076 w1084 w1092] -> w499
      tunnel: [w522 w563 w585 w598 w608 w648 w693 w734 w762 w812 w863 w899 w914 w954 w964 w983 w991 w1010 w1019 w1038 w1048 w1067 w1074 w1085 w1091] -> w493
      tunnel: w497 -> [w523 w560 w582 w598 w609 w646 w694 w734 w762 w812 w863 w899 w915 w954 w965 w983 w992 w1010 w1020 w1038 w1049 w1067 w1077 w1085 w1091]
      tunnel: [_ w548 _ _ w606 w627 w700 w729 _ _ _ w897 w923 _ w962 _ w990 _ w1018 _ w1046 _ _ _ _] -> w495
      tunnel: [_ w555 _ _ w605 w628 w699 w730 _ _ _ w896 w922 _ w961 _ w989 _ w1017 _ w1045 _ _ _ _] -> w494
      tunnel: [_ w531 _ _ w604 w626 w691 w728 _ _ _ w895 w920 _ w960 _ w988 _ w1016 _ w1044 _ _ _ _] -> w492
      tunnel: [_ w531 _ _ w604 _ w691 _ _ _ _ _ TRUE _ _ _ _ _ _ _ _ _ _ _ _] -> w491
      tunnel: [_ _ _ _ _ _ _ w728 _ _ _ w895 _ _ _ _ _ _ _ _ _ _ _ _ _] -> w486
      tunnel: [_ _ _ _ w604 _ _ _ _ _ _ _ _ w953 w960 w981 w988 w1009 w1016 w1037 w1044 _ _ _ _] -> w484
      tunnel: [_ _ _ _ w604 _ _ _ _ _ _ _ _ _ _ w981 w988 _ _ w1037 w1044 _ _ _ _] -> w483
      tunnel: [_ _ _ _ _ _ _ _ _ _ _ _ _ _ _ w981 w988 _ _ w1037 w1044 _ _ _ _] -> w482
      tunnel: w479 -> [_ w534 _ _ _ _ _ _ _ _ _ _ _ _ _ _ _ _ _ _ _ _ _ _ _]
      tunnel: [FALSE ("DAQ Started") w534 FALSE ("DAQ Started") FALSE ("DAQ Started") w604 w626 w691 w728 TRUE ("DAQ Started") TRUE ("DAQ Started") TRUE ("DAQ Started") TRUE ("DAQ Started") w920 w953 w960 w981 w988 w1009 w1016 w1037 w1044 TRUE ("DAQ Started") TRUE ("DAQ Started") TRUE ("DAQ Started") TRUE ("DAQ Started")] -> w478
      tunnel: w476 -> [_ w559 w581 _ w607 _ w692 w727 w757 w795 w849 _ w913 _ w963 _ w995 _ w1021 _ w1047 _ _ _ _]
      tunnel: w472 -> [_ w554 _ _ w605 w629 w690 w730 _ w796 w839 w896 w912 _ w961 _ w989 _ w1017 _ w1045 _ _ _ _]
      tunnel: w469 -> [_ w547 _ _ w606 w635 w689 w729 _ w797 w838 w897 w911 _ w962 _ w990 _ w1018 _ w1046 _ _ _ _]
      tunnel: w466 -> [_ w543 _ _ _ w639 _ _ _ _ _ _ _ _ _ _ _ _ _ _ _ _ _ _ _]
      tunnel: w465 -> [_ w545 _ _ _ w638 w687 _ _ _ _ _ _ _ _ _ _ _ _ _ _ _ _ _ _]
      tunnel: w464 -> [_ w544 _ _ _ w632 _ _ _ _ _ _ _ _ _ _ _ _ _ _ _ _ _ _ _]
      tunnel: w463 -> [_ w552 _ _ _ w631 w686 _ _ _ _ _ _ _ _ _ _ _ _ _ _ _ _ _ _]
      tunnel: w462 -> [_ w541 _ _ _ w625 w688 _ _ _ _ _ w910 _ _ _ _ _ _ _ _ _ _ _ _]
      frame #0 {
        n333 = call "Init Mixed Mode Command.vi"() -> ("Command Data"=w519:T6)  [unwired: 1 in, 2 out]
        n334 = call "Mixed Mode Commands DAO.vi"(7:LBCB_Number."LBCB1" ("LBCB Selected"), "Mixed Mode Commands\n Datastore Actions"=DAO_Actions."Init" ("Mixed Mode Commands\n Datastore Actions")) -> ()  [unwired: 2 in, 8 out]
        n335 = Bundle By Name(cluster=w523, "Command"=Mixed_Mode_Command_Action."No Op", "Ramp Times"=cluster{"Initial":T27, "Iterative":T27} {"Initial"={"Ramp"=0.0, "Stab"=0.0, "Hold"=0.0}, "Iterative"={"Ramp"=0.0, "Stab"=0.0, "Hold"=0.0}}, "LBCB1"=w519, "LBCB2"=w519) -> (w522:T31)
        n336 = call "Stiffness Jacobian DAO.vi"("LBCB Number"=LBCB_Number."LBCB1" ("LBCB Selected"), "Actions"=Persistant_DAO_Actions."Init" ("Stiffness Jacobian Datastore Actions")) -> ()  [unwired: 3 in, 7 out]
        n337 = call "Convergence Status DAO.vi"("Actions"=Persistant_DAO_Actions."Init") -> ()  [unwired: 3 in, 8 out]
      }
      frame #1 {
        w531 = TRUE
        w542 = LBCB_Conversions_Actions."A2C" ("Conversion Type")
        n338 = Not(x=w534) -> (.not. x?=w532:bool)
        n339 = Equal?(x=w536, y=Mixed_Mode_Command_Action."Measure Initial Position") -> (x = y?=w539:bool)
        n340 = And(x=w532, y=w539) -> (x .and. y?=w533:bool)
        n341 = Select(t=Mixed_Mode_States."Start Initial Position", s=w533, f=Mixed_Mode_States."Idle" ("MixedModeStates")) -> (s? t:f=w537:T24)
        n342 = Unbundle By Name(w552) -> ("Motion Center"=w556:dbl[], "Transformation Matrix"=w557:dbl[][])
        n343 = Unbundle By Name(w545) -> ("Motion Center"=w551:dbl[], "Transformation Matrix"=w550:dbl[][])
        n344 = Dequeue Element(queue=w565, timeout in ms (-1)=w559) -> (queue out=w564:refnum<queue>, element=w561:T31, timed out?=w562:bool)  [unwired: 1 in, 1 out]
        n345 = Equal?(x=Mixed_Mode_Command_Action."Start Command", y=w536) -> (x = y?=w567:bool)
        n346 = Select(t=w560, s=w562, f=w561) -> (s? t:f=w563:T31)
        n347 = Select(t=Mixed_Mode_States."Start Initial Ramp" ("MixedModeStates"), s=w567, f=w537) -> (s? t:f=w569:T24)
        n348 = Unbundle By Name(w554) -> ("Act Cmd"=w558:dbl[])
        n349 = Unbundle By Name(w547) -> ("Act Cmd"=w549:dbl[])
        n350 = call "LBCB_Conversions.vi"("Transformation Matrix"=w550, "Type"=w543, "Motion Center"=w551, "Conversion Type"=w542, "Input"=w549) -> ("Output"=w546:dbl[])  [unwired: 3 in, 3 out]
        n351 = case shown="\"2\"" w541 {
          tunnel: w558 -> [w573 w579]
          tunnel: w557 -> [_ w578]
          tunnel: w556 -> [_ w577]
          tunnel: [w573 w576] -> w553
          tunnel: w544 -> [_ w575]
          tunnel: w542 -> [_ w574]
          frame #0 {
          }
          frame #1 {
            n352 = call "LBCB_Conversions.vi"("Transformation Matrix"=w578, "Type"=w575, "Motion Center"=w577, "Conversion Type"=w574, "Input"=w579) -> ("Output"=w576:dbl[])  [unwired: 3 in, 3 out]
          }
        }
        n353 = Bundle By Name(cluster=w547, "Cart Cmd"=w546) -> (w548:T10)
        n354 = Bundle By Name(cluster=w554, "Cart Cmd"=w553) -> (w555:T10)
      }
      frame #2 {
        n355 = Dequeue Element(queue=w587, timeout in ms (-1)=w581) -> (queue out=w586:refnum<queue>, element=w583:T31, timed out?=w584:bool)  [unwired: 1 in, 1 out]
        n356 = Equal?(x=Mixed_Mode_Command_Action."Start Acquisition", y=w593) -> (x = y?=w589:bool)
        n357 = Select(t=w582, s=w584, f=w583) -> (s? t:f=w585:T31)
        n358 = Select(t=Mixed_Mode_States."Idle" ("MixedModeStates"), s=w589, f=Mixed_Mode_States."Wait For DAQ" ("MixedModeStates")) -> (s? t:f=w592:T24)
      }
      frame #3 {
        n359 = Unbundle By Name(w598) -> ("Ramp Times.Initial"=w597:T27)
      }
      frame #4 {
        w604 = TRUE
        n360 = Unbundle By Name(w620) -> ("Hold"=w616:dbl)
        n361 = Divide(x=w617, y=u64 1000) -> (x/y=w619:dbl)
        n362 = Greater?(x=w619, y=w616) -> (0:w615:bool)
        n363 = Dequeue Element(queue=w611, timeout in ms (-1)=w607) -> (queue out=w610:refnum<queue>, element=w612:T31, timed out?=w613:bool)  [unwired: 1 in, 1 out]
        n364 = Select(t=w609, s=w613, f=w612) -> (s? t:f=w608:T31)
        n365 = Select(t=Mixed_Mode_States."Done" ("MixedModeStates"), s=w615, f=Mixed_Mode_States."Initial Position") -> (s? t:f=w623:T24)
      }
      frame #5 {
        w626 = TRUE ("DAQ Started")
        w630 = LBCB_Conversions_Actions."A2C" ("Conversion Type")
        w640 = DAO_Actions."Set" ("Mixed Mode Commands\n Datastore Actions")
        n366 = Unbundle By Name(w646) -> ("Ramp Times.Initial"=w645:T27, "LBCB1"=w644:T6, "LBCB2"=w643:T6)
        n367 = Unbundle By Name(w643) -> ("Command Type"=w657:enum16{"<None>", "Displacement", "Force"}[])
        n368 = case shown="\"2\"" w625 {
          tunnel: w643 -> [w667 w679]
          tunnel: [w667 w678] -> w641
          tunnel: w640 -> [_ w677]
          tunnel: w632 -> [_ w676]
          tunnel: w631 -> [_ w675]
          tunnel: w630 -> [_ w671]
          tunnel: w629 -> [w666 w669]
          tunnel: [w666 w668] -> w628
          frame #0 {
          }
          frame #1 {
            n369 = Unbundle By Name(w675) -> ("Motion Center"=w674:dbl[], "Transformation Matrix"=w673:dbl[][])
            n370 = Unbundle By Name(w669) -> ("Act Cmd"=w672:dbl[])
            n371 = call "LBCB_Conversions.vi"("Transformation Matrix"=w673, "Type"=w676, "Motion Center"=w674, "Conversion Type"=w671, "Input"=w672) -> ("Output"=w670:dbl[])  [unwired: 3 in, 3 out]
            n372 = Bundle By Name(cluster=w669, "Cart Cmd"=w670) -> (w668:T10)
            n373 = call "Mixed Mode Commands DAO.vi"(7:LBCB_Number."LBCB2" ("LBCB Selected"), 9:w668, "Current Target In"=w679, "Mixed Mode Commands\n Datastore Actions"=w677) -> ("Current Target"=w678:T6[])  [unwired: 1 in, 6 out]
          }
        }
        n374 = Unbundle By Name(w644) -> ("Command Type"=w658:enum16{"<None>", "Displacement", "Force"}[])
        n375 = Unbundle By Name(w638) -> ("Motion Center"=w637:dbl[], "Transformation Matrix"=w636:dbl[][])
        n376 = Bundle By Name(cluster=w646, "Command"=Mixed_Mode_Command_Action."No Op") -> (w648:T31)
        n377 = for {
          tunnel: w658 -> [w685] mode=indexing
          tunnel: w657 -> [w684] mode=indexing
          tunnel: [w683] -> w656 mode=indexing
          tunnel: [w682] -> w655 mode=indexing
          w681 = enum16{"<None>", "Displacement", "Force"}."Displacement" ("x")
          n378 = Equal?(x=w681, y=w684) -> (x = y?=w682:bool)
          n379 = Equal?(x=w681, y=w685) -> (x = y?=w683:bool)
        }
        n380 = Unbundle By Name(w645) -> ("Ramp"=w665:dbl)
        n381 = Equal To 0?(x=w665) -> (x = 0?=w664:bool)
        n382 = Unbundle By Name(w635) -> ("Act Cmd"=w634:dbl[])
        n383 = call "LBCB_Conversions.vi"("Transformation Matrix"=w636, "Type"=w639, "Motion Center"=w637, "Conversion Type"=w630, "Input"=w634) -> ("Output"=w633:dbl[])  [unwired: 3 in, 3 out]
        n384 = Bundle By Name(cluster=w635, "Cart Cmd"=w633) -> (w627:T10)
        n385 = Build Array (concatenate)(w656, w655) -> (w654:bool[])
        n386 = call "Mixed Mode Commands DAO.vi"(7:LBCB_Number."LBCB1" ("LBCB Selected"), 9:w627, "Current Target In"=w644, "Mixed Mode Commands\n Datastore Actions"=w640) -> ("Current Target"=w642:T6[])  [unwired: 1 in, 6 out]
        n387 = Or Array Elements(Boolean array=w654) -> (logical OR=w650:bool)
        n388 = local write "L1 Current Target"(w642) -> ()
        n389 = Select(t=Mixed_Mode_States."Run Initial Ramp" ("MixedModeStates"), s=w650, f=Mixed_Mode_States."Start Iterative Stage" ("MixedModeStates")) -> (s? t:f=w653:T24)
        n390 = Select(t=Mixed_Mode_States."Idle" ("MixedModeStates"), s=w664, f=w653) -> (s? t:f=w662:T24)
        n391 = local write "L2 Current Target"(w641) -> ()
      }
      frame #6 {
        w691 = TRUE
        n392 = Unbundle By Name(w694) -> ("LBCB1.Space"=w710:T7)
        n393 = local read "LBCB 2 Setting"() -> (w708:T15)
        n394 = local read "LBCB 1 Setting"() -> (w709:T15)
        n395 = Unbundle By Name(w709) -> ("Type"=w707:T17)
        n396 = call "Ramp Time Completions.vi"("Current Ramp Time"=w714, "Initial"=w712) -> ("Still in Ramp"=w705:bool, "Fraction\nCompleted"=w704:dbl)
        n397 = Unbundle By Name(w708) -> ("Type"=w706:T17)
        n398 = case shown="False" w705 {
          tunnel: w704 -> [w720 _]
          tunnel: [Mixed_Mode_States."Run Initial Ramp" ("MixedModeStates") Mixed_Mode_States."Start Iterative Stage" ("MixedModeStates")] -> w701
          tunnel: [w716 w722] -> w703
          tunnel: [w715 w723] -> w702
          frame #0 {
            n399 = call "Calculate Ramp Displacements.vi"(2:LBCB_Number."LBCB1" ("LBCB Selected"), "Ramp Time"=w720) -> ("Target"=w716:T6[])  [unwired: 1 in]
            n400 = call "Calculate Ramp Displacements.vi"(2:LBCB_Number."LBCB2" ("LBCB Selected"), "Ramp Time"=w720) -> ("Target"=w715:T6[])  [unwired: 1 in]
          }
          frame #1 {
            w721 = DAO_Actions."Get" ("Mixed Mode Commands\n Datastore Actions")
            n401 = call "Mixed Mode Commands DAO.vi"(7:LBCB_Number."LBCB1" ("LBCB Selected"), "Mixed Mode Commands\n Datastore Actions"=w721) -> ("Current Target"=w722:T6[])  [unwired: 2 in, 7 out]
            n402 = call "Mixed Mode Commands DAO.vi"(7:LBCB_Number."LBCB2" ("LBCB Selected"), "Mixed Mode Commands\n Datastore Actions"=w721) -> ("Current Target"=w723:T6[])  [unwired: 2 in, 7 out]
          }
        }
        n403 = Dequeue Element(queue=w696, timeout in ms (-1)=w692) -> (queue out=w695:refnum<queue>, element=w698:T31, timed out?=w697:bool)  [unwired: 1 in, 1 out]
        n404 = Select(t=w694, s=w697, f=w698) -> (s? t:f=w693:T31)
        n405 = call "MM Command to Cntrl Loop Actuator In.vi"("Space"=w710, "Target"=w703, 2:w702, "Prev  Cmd"=w689, "Number of\nLBCBs In"=w688, "LBCB Type"=w707, 11:w706, "Position"=w687, 13:w686, 14:w690) -> ("Cmd Out"=w700:T10[], 10:w699)  [unwired: 1 in, 3 out]
      }
      frame #7 {
        w728 = TRUE
        w733 = Persistant_DAO_Actions."Set" ("Actions")
        w747 = T23 {"IsConverged"=[], "Force Errors"=[], "MaxForceDiffIndex"=0} ("Convergence Status Out")
        n406 = Unbundle By Name(w734) -> ("LBCB2.Command Type"=w749:enum16{"<None>", "Displacement", "Force"}[])
        n407 = Unbundle By Name(w734) -> ("LBCB1.Command Type"=w750:enum16{"<None>", "Displacement", "Force"}[])
        n408 = Wait Until Next ms Multiple(millisecond multiple=w727) -> ()  [unwired: 1 out]
        n409 = for {
          tunnel: w750 -> [w752] mode=indexing
          tunnel: w749 -> [w753] mode=indexing
          tunnel: [w756] -> w744 mode=indexing
          tunnel: [w755] -> w743 mode=indexing
          w754 = enum16{"<None>", "Displacement", "Force"}."Force" ("x")
          n410 = Not Equal?(x=w754, y=w753) -> (x != y?=w755:bool)
          n411 = Not Equal?(x=w754, y=w752) -> (x != y?=w756:bool)
        }
        n412 = Initialize Array(0.0 ("element"), 6 ("dimension size")) -> (w739:dbl[])
        n413 = Bundle By Name(cluster=w747, "IsConverged"=w743, "Force Errors"=w739) -> (w746:T23)
        n414 = Bundle By Name(cluster=w747, "IsConverged"=w744, "Force Errors"=w739) -> (w745:T23)
        n415 = call "Convergence Status DAO.vi"("Convergence Status In"=w745, "LBCB Selected"=LBCB_Number."LBCB1", "Actions"=w733) -> ("Convergence Status Out"=w732:T23)  [unwired: 1 in, 7 out]
        n416 = call "Convergence Status DAO.vi"("Convergence Status In"=w746, "LBCB Selected"=LBCB_Number."LBCB2", "Actions"=w733) -> ("Convergence Status Out"=w731:T23)  [unwired: 1 in, 7 out]
        n417 = local write "L2 Convergence Status"(w731) -> ()
        n418 = local write "L1 Convergence Status"(w732) -> ()
      }
      frame #8 {
        w760 = DAO_Actions."Get" ("Mixed Mode Commands\n Datastore Actions")
        w759 = LBCB_Number."LBCB2" ("LBCB Selected")
        w758 = LBCB_Number."LBCB1" ("LBCB Selected")
        w783 = Persistant_DAO_Actions."Get" ("Mixed Mode \n Datastore Actions")
        w784 = Persistant_DAO_Actions."Set" ("Mixed Mode \n Datastore Actions")
        n419 = local read "L1 Measurements"() -> (w769:T21)
        n420 = local read "L2 Measurements"() -> (w768:T21)
        n421 = call "Mixed Mode Commands DAO.vi"(7:w759, "Mixed Mode Commands\n Datastore Actions"=w760) -> ("Current Target"=w770:T6[])  [unwired: 2 in, 7 out]
        n422 = call "Mixed Mode Commands DAO.vi"(7:w758, "Mixed Mode Commands\n Datastore Actions"=w760) -> ("Current Target"=w771:T6[])  [unwired: 2 in, 7 out]
        n423 = local read "L1 Force Error Range"() -> (w765:dbl[])
        n424 = Wait Until Next ms Multiple(millisecond multiple=w757) -> ()  [unwired: 1 out]
        n425 = Unbundle By Name(w768) -> ("Cart Forces"=w766:dbl[])
        n426 = Unbundle By Name(w769) -> ("Cart Forces"=w767:dbl[])
        n427 = Equal?(x=Mixed_Mode_States."Start Iterative Stage" ("t"), y=w774) -> (x = y?=w773:bool)
        n428 = local read "L2 Force Error Range"() -> (w764:dbl[])
        n429 = call "Convergence Status DAO.vi"("LBCB Selected"=w758, "Actions"=w783) -> ("Convergence Status Out"=w781:T23)  [unwired: 2 in, 7 out]
        n430 = call "Convergence Status DAO.vi"("LBCB Selected"=w759, "Actions"=w783) -> ("Convergence Status Out"=w782:T23)  [unwired: 2 in, 7 out]
        n431 = call "Convergence Check.vi"("Forces Error \nTolerances"=w765, "Command Data"=w771, "Cart\nForces"=w767, "Mixed Mode Convergence Status In"=w781) -> ("Mixed Mode Convergence Status Out"=w786:T23)  [unwired: 1 in, 6 out]
        n432 = call "Convergence Check.vi"("Forces Error \nTolerances"=w764, "Command Data"=w770, "Cart\nForces"=w766, "Mixed Mode Convergence Status In"=w782) -> ("Mixed Mode Convergence Status Out"=w785:T23)  [unwired: 1 in, 6 out]
        n433 = Unbundle By Name(w785) -> ("IsConverged"=w793:bool[])
        n434 = call "Convergence Status DAO.vi"("Convergence Status In"=w786, "LBCB Selected"=w758, "Actions"=w784) -> ("Convergence Status Out"=w779:T23)  [unwired: 1 in, 7 out]
        n435 = Unbundle By Name(w786) -> ("IsConverged"=w794:bool[])
        n436 = call "Convergence Status DAO.vi"("Convergence Status In"=w785, "LBCB Selected"=w759, "Actions"=w784) -> ("Convergence Status Out"=w780:T23)  [unwired: 1 in, 7 out]
        n437 = local write "L1 Convergence Status"(w779) -> ()
        n438 = local write "L2 Convergence Status"(w780) -> ()
        n439 = Select(t=Mixed_Mode_States."Update Command", s=w773, f=Mixed_Mode_States."Update Stiffness Jacobian") -> (s? t:f=w777:T24)
        n440 = Build Array (concatenate)(w794, w793) -> (w792:bool[])
        n441 = And Array Elements(Boolean array=w792) -> (logical AND=w791:bool)
        n442 = Select(t=Mixed_Mode_States."Start Stabilize" ("MixedModeStates"), s=w791, f=w777) -> (s? t:f=w789:T24)
      }
      frame #9 {
        w826 = T5 {"Displacements"=[], "Forces"=[]} ("Increments")
        w828 = LBCB_Number."LBCB2" ("LBCB Selected")
        w829 = LBCB_Number."LBCB1" ("LBCB Selected")
        n443 = local read "L2 Measurements"() -> (w799:T21)
        n444 = local read "L1 Measurements"() -> (w801:T21)
        n445 = local write "L2 Previous Target"(w808) -> ()
        n446 = Unbundle By Name(w808) -> ("Displacements"=w817:dbl[], "Forces"=w816:dbl[])
        n447 = local write "L1 Previous Target"(w807) -> ()
        n448 = Unbundle By Name(w807) -> ("Displacements"=w821:dbl[], "Forces"=w819:dbl[])
        n449 = Unbundle By Name(w801) -> ("Cart Forces"=w802:dbl[])
        n450 = call "Calculated Stiffness Jacobian.vi"("LBCB Number"=w829, "Actions"=Persistant_DAO_Actions."Get" ("Stiffness Jacobian Datastore Actions")) -> ("Stiffness Jacobian Out"=w836:T22)  [unwired: 2 in, 7 out]
        n451 = Unbundle By Name(w796) -> ("Cart Cmd"=w798:dbl[])
        n452 = Unbundle By Name(w799) -> ("Cart Forces"=w800:dbl[])
        n453 = call "Calculated Stiffness Jacobian.vi"("LBCB Number"=w828, "Actions"=Persistant_DAO_Actions."Get" ("Stiffness Jacobian Datastore Actions")) -> ("Stiffness Jacobian Out"=w832:T22)  [unwired: 2 in, 7 out]
        n454 = Wait Until Next ms Multiple(millisecond multiple=w795) -> ()  [unwired: 1 out]
        n455 = Unbundle By Name(w797) -> ("Cart Cmd"=w803:dbl[])
        n456 = local read "L1 Convergence Status"() -> (w805:T23)
        n457 = Subtract(x=w802, y=w819) -> (x-y=w818:dbl[])
        n458 = Subtract(x=w800, y=w816) -> (x-y=w814:dbl[])
        n459 = Subtract(x=w798, y=w817) -> (x-y=w815:dbl[])
        n460 = Subtract(x=w803, y=w821) -> (x-y=w820:dbl[])
        n461 = local read "L2 Convergence Status"() -> (w804:T23)
        n462 = Bundle By Name(cluster=w826, "Displacements"=w815, "Forces"=w814) -> (w824:T5)
        n463 = call "Update Stiffness Jacobian.vi"("Mixed Mode Convergence Status In"=w804, "Increments"=w824, "Stiffness Jacobian In"=w832) -> ("Stiffness Jacobian Out"=w831:T22)  [unwired: 8 out]
        n464 = Bundle By Name(cluster=w826, "Displacements"=w820, "Forces"=w818) -> (w825:T5)
        n465 = call "Calculated Stiffness Jacobian.vi"("Stiffness Jacobian In"=w831, "LBCB Number"=w828, "Actions"=Persistant_DAO_Actions."Set" ("Stiffness Jacobian Datastore Actions")) -> ("Stiffness Jacobian Out"=w810:T22)  [unwired: 1 in, 7 out]
        n466 = local write "L2 Stiffness Jacobian"(w810) -> ()
        n467 = call "Update Stiffness Jacobian.vi"("Mixed Mode Convergence Status In"=w805, "Increments"=w825, "Stiffness Jacobian In"=w836) -> ("Stiffness Jacobian Out"=w835:T22)  [unwired: 8 out]
        n468 = call "Calculated Stiffness Jacobian.vi"("Stiffness Jacobian In"=w835, "LBCB Number"=w829, "Actions"=Persistant_DAO_Actions."Set" ("Stiffness Jacobian Datastore Actions")) -> ("Stiffness Jacobian Out"=w809:T22)  [unwired: 1 in, 7 out]
        n469 = local write "L1 Stiffness Jacobian"(w809) -> ()
      }
      frame #10 {
        w860 = T5 {"Displacements"=[], "Forces"=[]} ("Cartesian  Data")
        w844 = DAO_Actions."Set" ("Mixed Mode Commands\n Datastore Actions")
        w854 = DAO_Actions."Get" ("Mixed Mode Commands\n Datastore Actions")
        w843 = LBCB_Number."LBCB2" ("LBCB Selected")
        w848 = LBCB_Number."LBCB1" ("LBCB Selected")
        n470 = local read "L2 Measurements"() -> (w861:T21)
        n471 = local read "L1 Measurements"() -> (w862:T21)
        n472 = Unbundle By Name(w838) -> ("Cart Cmd"=w859:dbl[])
        n473 = Unbundle By Name(w839) -> ("Cart Cmd"=w857:dbl[])
        n474 = Unbundle By Name(w861) -> ("Cart Forces"=w856:dbl[])
        n475 = Unbundle By Name(w862) -> ("Cart Forces"=w858:dbl[])
        n476 = Wait Until Next ms Multiple(millisecond multiple=w849) -> ()  [unwired: 1 out]
        n477 = Bundle By Name(cluster=w860, "Displacements"=w859, "Forces"=w858) -> (w840:T5)
        n478 = Bundle By Name(cluster=w860, "Displacements"=w857, "Forces"=w856) -> (w841:T5)
        n479 = call "Mixed Mode Commands DAO.vi"(7:w843, "Mixed Mode Commands\n Datastore Actions"=w854) -> ("Current Target"=w866:T6[])  [unwired: 3 in, 6 out]
        n480 = call "Convergence Status DAO.vi"("LBCB Selected"=w843, "Actions"=w854) -> ("Convergence Status Out"=w869:T23)  [unwired: 2 in, 7 out]
        n481 = call "Convergence Status DAO.vi"("LBCB Selected"=w848, "Actions"=w854) -> ("Convergence Status Out"=w871:T23)  [unwired: 2 in, 7 out]
        n482 = Unbundle By Name(w869) -> ("MaxForceDiffIndex"=w868:i32, "IsConverged"=w851:bool[])
        n483 = Unbundle By Name(w871) -> ("MaxForceDiffIndex"=w870:i32, "IsConverged"=w853:bool[])
        n484 = call "Mixed Mode Commands DAO.vi"(7:w848, "Mixed Mode Commands\n Datastore Actions"=w854) -> ("Current Target"=w867:T6[])  [unwired: 2 in, 7 out]
        n485 = And Array Elements(Boolean array=w853) -> (logical AND=w852:bool)
        n486 = And Array Elements(Boolean array=w851) -> (logical AND=w850:bool)
        n487 = case shown="True" w850 {
          tunnel: w868 -> [w881 _]
          tunnel: w866 -> [w880 w884]
          tunnel: w843 -> [w876 _]
          tunnel: w841 -> [w879 _]
          tunnel: [w875 w883] -> w845
          tunnel: w839 -> [_ w882]
          frame #0 {
            n488 = local read "L2 Max Increment"() -> (w877:dbl[])
            n489 = local read "L2 Jacobian Gain"() -> (w878:dbl[])
            n490 = call "Update Iterative Command.vi"("Maximum Displacement\nIncrement"=w877, "Jacobian Gain"=w878, "LBCB Selected"=w876, "Max Force Diff Index"=w881, "Current  Data In"=w879, "Target  Command Data In"=w880) -> ("Updated  Command Data Out"=w875:T6)  [unwired: 5 out]
          }
          frame #1 {
            n491 = call "Command Data 2 Control Target.vi"("Command\nData"=w882, "Current Target"=w884) -> ("Output"=w883:T6)  [unwired: 9 out]
          }
        }
        n492 = case shown="True" w852 {
          tunnel: [w885 w893] -> w847
          tunnel: w870 -> [w891 _]
          tunnel: w867 -> [w890 w894]
          tunnel: w848 -> [w886 _]
          tunnel: w840 -> [w889 _]
          tunnel: w838 -> [_ w892]
          frame #0 {
            n493 = local read "L1 Max Increment"() -> (w888:dbl[])
            n494 = local read "L1 Jacobian Gain"() -> (w887:dbl[])
            n495 = call "Update Iterative Command.vi"("Maximum Displacement\nIncrement"=w888, "Jacobian Gain"=w887, "LBCB Selected"=w886, "Max Force Diff Index"=w891, "Current  Data In"=w889, "Target  Command Data In"=w890) -> ("Updated  Command Data Out"=w885:T6)  [unwired: 5 out]
          }
          frame #1 {
            n496 = call "Command Data 2 Control Target.vi"("Command\nData"=w892, "Current Target"=w894) -> ("Output"=w893:T6)  [unwired: 9 out]
          }
        }
        n497 = call "Mixed Mode Commands DAO.vi"(7:w848, 9:w838, "Current Target In"=w847, "Mixed Mode Commands\n Datastore Actions"=w844) -> ("Current Target"=w846:T6[])  [unwired: 1 in, 6 out]
        n498 = local write "L1 Iterative Target"(w846) -> ()
        n499 = call "Mixed Mode Commands DAO.vi"(7:w843, 9:w839, "Current Target In"=w845, "Mixed Mode Commands\n Datastore Actions"=w844) -> ("Current Target"=w842:T6[])  [unwired: 1 in, 6 out]
        n500 = local write "L2 Iterative Target"(w842) -> ()
      }
      frame #11 {
        w895 = TRUE
        n501 = Unbundle By Name(w899) -> ("Ramp Times.Iterative"=w909:T27)
        n502 = Unbundle By Name(w909) -> ("Ramp"=w904:dbl)
        n503 = Equal To 0?(x=w904) -> (x = 0?=w905:bool)
        n504 = Select(t=u32 1, s=w905, f=w904) -> (s? t:f=w903:dbl)
        n505 = Bundle By Name(cluster=w909, "Ramp"=w903) -> (w906:T27)
      }
      frame #12 {
        w920 = TRUE
        n506 = local read "LBCB 2 Setting"() -> (w926:T15)
        n507 = local read "LBCB 1 Setting"() -> (w927:T15)
        n508 = Unbundle By Name(w927) -> ("Type"=w925:T17)
        n509 = Unbundle By Name(w926) -> ("Type"=w924:T17)
        n510 = call "Ramp Time Completions.vi"("Current Ramp Time"=w937, "Initial"=w935) -> ("Still in Ramp"=w938:bool, "Fraction\nCompleted"=w939:dbl)
        n511 = case shown="True" w938 {
          tunnel: w939 -> [_ w952]
          tunnel: [Mixed_Mode_States."Start Iterative Stabilize" ("MixedModeStates") Mixed_Mode_States."Run Iterative Ramp" ("MixedModeStates")] -> w933
          tunnel: [w942 w947] -> w932
          tunnel: [w941 w946] -> w931
          frame #0 {
            w940 = DAO_Actions."Get" ("Mixed Mode Commands\n Datastore Actions")
            n512 = call "Mixed Mode Commands DAO.vi"(7:LBCB_Number."LBCB1" ("LBCB Selected"), "Mixed Mode Commands\n Datastore Actions"=w940) -> ("Current Target"=w942:T6[])  [unwired: 2 in, 7 out]
            n513 = call "Mixed Mode Commands DAO.vi"(7:LBCB_Number."LBCB2" ("LBCB Selected"), "Mixed Mode Commands\n Datastore Actions"=w940) -> ("Current Target"=w941:T6[])  [unwired: 2 in, 7 out]
          }
          frame #1 {
            w948 = TRUE ("Iterative\nRamp")
            n514 = call "Calculate Ramp Displacements.vi"("Iterative\nRamp"=w948, 2:LBCB_Number."LBCB1" ("LBCB Selected"), "Ramp Time"=w952) -> ("Target"=w947:T6[])
            n515 = call "Calculate Ramp Displacements.vi"("Iterative\nRamp"=w948, 2:LBCB_Number."LBCB2" ("LBCB Selected"), "Ramp Time"=w952) -> ("Target"=w946:T6[])
          }
        }
        n516 = Dequeue Element(queue=w917, timeout in ms (-1)=w913) -> (queue out=w916:refnum<queue>, element=w918:T31, timed out?=w919:bool)  [unwired: 1 in, 1 out]
        n517 = Unbundle By Name(w915) -> ("LBCB1.Space"=w930:T7)
        n518 = local read "L2 Position"() -> (w928:T20)
        n519 = local read "L1  Position"() -> (w929:T20)
        n520 = Select(t=w915, s=w919, f=w918) -> (s? t:f=w914:T31)
        n521 = call "MM Command to Cntrl Loop Actuator In.vi"("Space"=w930, "Target"=w932, 2:w931, "Prev  Cmd"=w911, "Number of\nLBCBs In"=w910, "LBCB Type"=w925, 11:w924, "Position"=w929, 13:w928, 14:w912) -> ("Cmd Out"=w923:T10[], 10:w922)  [unwired: 1 in, 3 out]
      }
      frame #13 {
        w953 = TRUE
        n522 = Unbundle By Name(w954) -> ("Ramp Times.Iterative"=w957:T27)
      }
      frame #14 {
        w960 = TRUE
        n523 = Unbundle By Name(w971) -> ("Stab"=w976:dbl)
        n524 = Divide(x=w973, y=u64 1000) -> (x/y=w975:dbl)
        n525 = Greater?(x=w975, y=w976) -> (0:w972:bool)
        n526 = Dequeue Element(queue=w967, timeout in ms (-1)=w963) -> (queue out=w966:refnum<queue>, element=w968:T31, timed out?=w969:bool)  [unwired: 1 in, 1 out]
        n527 = Select(t=w965, s=w969, f=w968) -> (s? t:f=w964:T31)
        n528 = Select(t=Mixed_Mode_States."Start Iterative Holding" ("MixedModeStates"), s=w972, f=Mixed_Mode_States."Iterative Stabilize" ("MixedModeStates")) -> (s? t:f=w977:T24)
      }
      frame #15 {
        w981 = TRUE
      }
      frame #16 {
        w988 = TRUE
        n529 = Unbundle By Name(w1004) -> ("Hold"=w1000:dbl)
        n530 = Divide(x=w1001, y=u64 1000) -> (x/y=w1003:dbl)
        n531 = Greater?(x=w1003, y=w1000) -> (0:w999:bool)
        n532 = Dequeue Element(queue=w994, timeout in ms (-1)=w995) -> (queue out=w993:refnum<queue>, element=w996:T31, timed out?=w997:bool)  [unwired: 1 in, 1 out]
        n533 = Select(t=w992, s=w997, f=w996) -> (s? t:f=w991:T31)
        n534 = Select(t=Mixed_Mode_States."Convergence Check" ("MixedModeStates"), s=w999, f=Mixed_Mode_States."Iterative Holding") -> (s? t:f=w1007:T24)
      }
      frame #17 {
        w1009 = TRUE
        n535 = Unbundle By Name(w1010) -> ("Ramp Times.Initial"=w1013:T27)
      }
      frame #18 {
        w1016 = TRUE
        n536 = Unbundle By Name(w1027) -> ("Stab"=w1032:dbl)
        n537 = Divide(x=w1029, y=u64 1000) -> (x/y=w1031:dbl)
        n538 = Dequeue Element(queue=w1023, timeout in ms (-1)=w1021) -> (queue out=w1022:refnum<queue>, element=w1024:T31, timed out?=w1025:bool)  [unwired: 1 in, 1 out]
        n539 = Greater?(x=w1031, y=w1032) -> (0:w1028:bool)
        n540 = Select(t=w1020, s=w1025, f=w1024) -> (s? t:f=w1019:T31)
        n541 = Select(t=Mixed_Mode_States."Start Hold" ("MixedModeStates"), s=w1028, f=Mixed_Mode_States."Stabilize" ("MixedModeStates")) -> (s? t:f=w1033:T24)
      }
      frame #19 {
        w1037 = TRUE
      }
      frame #20 {
        w1044 = TRUE
        n542 = Unbundle By Name(w1060) -> ("Hold"=w1056:dbl)
        n543 = Divide(x=w1057, y=u64 1000) -> (x/y=w1059:dbl)
        n544 = Greater?(x=w1059, y=w1056) -> (0:w1055:bool)
        n545 = Dequeue Element(queue=w1051, timeout in ms (-1)=w1047) -> (queue out=w1050:refnum<queue>, element=w1052:T31, timed out?=w1053:bool)  [unwired: 1 in, 1 out]
        n546 = Select(t=w1049, s=w1053, f=w1052) -> (s? t:f=w1048:T31)
        n547 = Select(t=Mixed_Mode_States."Done" ("MixedModeStates"), s=w1055, f=Mixed_Mode_States."Holding") -> (s? t:f=w1063:T24)
      }
      frame #21 {
        n548 = Wait Until Next ms Multiple(millisecond multiple=u32 100) -> ()  [unwired: 1 out]
      }
      frame #22 {
        n549 = Bundle By Name(cluster=w1077, "Command"=Mixed_Mode_Command_Action."No Op") -> (w1074:T31)
        n550 = Wait Until Next ms Multiple(millisecond multiple=u32 200) -> ()  [unwired: 1 out]
      }
      frame #23 {
      }
      frame #24 {
      }
    }
    "Collecting DAQ Samples" <- w478
    n551 = Not Equal?(x=w487, y=w503) -> (x != y?=w504:bool)
    n552 = case shown="True" w492 {
      tunnel: w495 -> [_ w1137]
      tunnel: w494 -> [_ w1136]
      tunnel: w491 -> [_ w1135]
      tunnel: w490 -> [w1109 w1130]
      tunnel: w489 -> [w1108 w1128]
      tunnel: [w1108 w1127] -> w488
      tunnel: [w1109 w1129] -> w477
      tunnel: w486 -> [_ w1124]
      tunnel: w475 -> [_ w1119]
      tunnel: w463 -> [_ w1116]
      tunnel: w464 -> [_ w1115]
      tunnel: w465 -> [_ w1114]
      tunnel: w466 -> [_ w1113]
      frame #0 {
      }
      frame #1 {
        w1110 = TRUE ("Convert\nCart\nMeasurements")
        # "Collect Measurements and Check Limits"
        n553 = local read "L1  Limits"() -> (w1117:T18)
        n554 = local read "L2 Limits"() -> (w1118:T18)
        n555 = local read "L2 Measurements"() -> (w1111:T21)
        n556 = local read "L1 Measurements"() -> (w1112:T21)
        n557 = local read "L2 Actuator Meas. Disp & Forces"() -> (w1140:dbl[])
        n558 = local read "L1 Actuator Meas. Disp & Forces"() -> (w1139:dbl[])
        n559 = case shown="\"2\"" w1119 {
          tunnel: [w1144 w1156] -> w1142
          tunnel: w1140 -> [_ w1155]
          tunnel: w1115 -> [_ w1154]
          tunnel: w1116 -> [_ w1153]
          tunnel: w1136 -> [_ w1152]
          tunnel: [w1145 w1151] -> w1134
          tunnel: [w1143 w1150] -> w1123
          tunnel: w1118 -> [_ w1148]
          tunnel: w1110 -> [_ w1147]
          tunnel: w1111 -> [_ w1146]
          frame #0 {
            n560 = call "Fake Actuator Measurements.vi"() -> ("Measurements"=w1143:T55, "Commands"=w1145:T10, "Within Limits"=w1144:T14)  [unwired: 13 out]
          }
          frame #1 {
            n561 = call "Collect Actuator Measurements.vi"("Actuator Meas. \nDisp & Forces"=w1155, "LBCB Number"=LBCB_Number."LBCB2", 2:w1147, "Commands In"=w1152, 7:w1146, "Limits"=w1148, "LBCB Position"=w1153, "Type"=w1154) -> ("Measurements Out"=w1150:T56, "Commands Out"=w1151:T10, "Within Limits"=w1156:T14)  [unwired: 1 in, 4 out]
          }
        }
        n562 = call "Collect Actuator Measurements.vi"("Actuator Meas. \nDisp & Forces"=w1139, "LBCB Number"=LBCB_Number."LBCB1", 2:w1110, "Commands In"=w1137, 7:w1112, "Limits"=w1117, "LBCB Position"=w1114, "Type"=w1113) -> ("Measurements Out"=w1121:T56, "Commands Out"=w1133:T10, "Within Limits"=w1141:T14)  [unwired: 1 in, 4 out]
        n563 = Unbundle By Name(w1121) -> ("Cart Forces"=w1120:dbl[])
        n564 = Unbundle By Name(w1133) -> ("Act Cmd"=w1132:dbl[], "Cart Cmd"=w1126:dbl[])
        n565 = Unbundle By Name(w1123) -> ("Cart Forces"=w1122:dbl[])
        n566 = Unbundle By Name(w1134) -> ("Act Cmd"=w1131:dbl[], "Cart Cmd"=w1125:dbl[])
        n567 = local write "L2 Measurements"(w1123) -> ()
        n568 = local write "L1 Commands"(w1133) -> ()
        n569 = local write "L2 Faults"(w1142) -> ()
        n570 = local write "L2 Commands"(w1134) -> ()
        n571 = local write "L1 Measurements"(w1121) -> ()
        n572 = case shown="True" w1124 {
          tunnel: w1130 -> [w1158 w1166]
          tunnel: [w1158 w1165] -> w1129
          tunnel: w1128 -> [w1157 w1164]
          tunnel: [w1157 w1163] -> w1127
          tunnel: w1126 -> [_ w1162]
          tunnel: w1125 -> [_ w1161]
          tunnel: w1122 -> [_ w1160]
          tunnel: w1120 -> [_ w1159]
          frame #0 {
          }
          frame #1 {
            # "Store for Stiffness\nJacobian Previous Target"
            n573 = Bundle By Name(cluster=w1166, "Displacements"=w1162, "Forces"=w1159) -> (w1165:T5)
            n574 = Bundle By Name(cluster=w1164, "Displacements"=w1161, "Forces"=w1160) -> (w1163:T5)
          }
        }
        n575 = local write "L1 Faults"(w1141) -> ()
        n576 = case shown="True" w1135 {
          tunnel: w1132 -> [_ w1168]
          tunnel: w1131 -> [_ w1167]
          frame #0 {
          }
          frame #1 {
            # "Send Cmds after Limit Check"
            n577 = local write "L1 Ctrl Loop In Actuator"(w1168) -> ()
            n578 = local write "L2 Ctrl Loop In Actuator"(w1167) -> ()
          }
        }
      }
    }
    n579 = case shown="False" w504 {
      tunnel: w507 -> [w1170 w1175]
      tunnel: [w1170 w1174] -> w506
      tunnel: w505 -> [w1169 w1173]
      tunnel: [w1169 w1172] -> w498
      tunnel: w487 -> [_ w1171]
      frame #0 {
      }
      frame #1 {
        n580 = Send Notification(notification=w1171, notifier=w1175, error in (no error)=w1173) -> (notifier out=w1174:refnum<notifier>, error out=w1172:errorcluster)
      }
    }
    n581 = flat-sequence {
      tunnel: w484 -> [w1105]
      tunnel: w483 -> [w1104]
      tunnel: w482 -> [w1098]
      tunnel: w477 -> [_]
      frame #0 {
        # "Hack job for\nRace Condition"
        n582 = local read "L1 PID Control"() -> (w1106:T8)
        n583 = local read "L2 PID Control"() -> (w1107:T8)
        n584 = local write "Hold Period"(w1104) -> ()
        n585 = local write "Averaging"(w1105) -> ()
        n586 = Unbundle By Name(w1106) -> ("I-Control"=w1100:bool, "Ctrl Mode"=w1099:bool)
        n587 = Unbundle By Name(w1107) -> ("I-Control"=w1103:bool, "Ctrl Mode"=w1102:bool)
        n588 = Compound Arithmetic op=AND(w1103, w1102, w1098) -> (w1101:bool)
        n589 = Compound Arithmetic op=AND(w1100, w1099, w1098) -> (w1097:bool)
        n590 = local write "L1 PID On"(w1101) -> ()
        n591 = local write "L2 PID On"(w1097) -> ()
      }
    }
    n592 = local read "App Running"() -> (w485:bool)
    n593 = local write "MixedModeStates"(w487) -> ()
    n594 = Not(x=w485) -> (.not. x?=w480:bool)
  }
  n595 = Initialize Array(0.0 ("element"), 6 ("dimension size")) -> (w41:dbl[])
  n596 = call "Autobalance Initial State DAO.vi"() -> ("autobalance\nfile"=w59:string, "Initial Values"=w63:T1[])  [unwired: 3 in, 7 out]
  n597 = Initialize Array(0.0 ("element"), 6 ("dimension size")) -> (w42:dbl[])
  n598 = local write "L2 Ctrl Loop In Actuator"(w42) -> ()
  n599 = call "Autobalance Initial State DAO.vi"() -> ("Initial Values"=w56:T1[])  [unwired: 3 in, 8 out]
  n600 = while {
    shift-right: [w1195] -> _
    shift-left: w41 -> [w1199]
    tunnel: w26 -> [w1198]
    shift-right: [w1190] -> _
    shift-left: w63 -> [w1193]
    tunnel: LBCB_Number."LBCB1" ("LBCB Number") -> [w1192]
    tunnel: [w1191] -> w51
    shift-right: [w1189] -> _
    shift-left: Autobalance_State."Init" ("Autobalance State Out") -> [w1188]
    shift-right: [w1187] -> _
    shift-left: _ -> [w1186]
    shift-right: [w1185] -> _
    shift-left: _ -> [w1184]
    tunnel: w11 -> [w1183]
    tunnel: w7 -> [w1182]
    stop <- w1191 stop-if-true
    # "LBCB 1 Control Loop"
    # "Cartesian\nCommand\nNo  Offset"
    # "Actuator Command"
    n601 = call "GetSamplingRate.vi"() -> ("Sampling"=w1197:i32)
    n602 = local read "L1 Ctrl Loop In Actuator"() -> (w1196:dbl[])
    n603 = local read "App Running"() -> (w1200:bool)
    n604 = local read "L1 Ctrl Loop State"() -> (w1201:T9)
    n605 = local write "L1 Control Rate"(w1197) -> ()
    n606 = Not(x=w1200) -> (.not. x?=w1191:bool)
    n607 = case shown="\"Autobalancing\"" w1201 {
      tunnel: w1197 -> [_ _ _ _ _ _ w1283]
      tunnel: [w1206 w1212 w1220 w1226 w1253 w1263 w1271] -> w1195
      tunnel: w1199 -> [w1206 w1212 w1220 _ _ w1263 w1268]
      tunnel: w1198 -> [w1207 w1213 w1221 w1233 w1252 w1264 w1282]
      tunnel: w1192 -> [_ _ _ w1227 w1251 _ w1281]
      tunnel: w1196 -> [_ _ _ _ _ _ w1269]
      tunnel: [w1205 w1211 w1219 w1231 w1246 w1262 w1278] -> w1185
      tunnel: [w1208 w1214 w1217 w1222 w1242 w1265 w1270] -> w1190
      tunnel: w1193 -> [w1208 w1214 _ w1223 w1243 w1265 w1270]
      tunnel: [w1204 w1210 Autobalance_State."Init" ("Autobalance State Out") w1225 w1249 w1261 w1267] -> w1189
      tunnel: w1188 -> [w1204 w1210 _ w1225 w1250 w1261 w1267]
      tunnel: [w1203 w1209 T2 TRUE ("InitialPosition? Out") w1224 w1247 w1260 w1266] -> w1187
      tunnel: w1186 -> [w1203 w1209 _ w1224 w1248 w1260 w1266]
      tunnel: w1184 -> [_ _ _ _ w1244 _ _]
      tunnel: w1183 -> [_ _ _ _ w1238 _ _]
      tunnel: w1182 -> [_ _ _ _ w1237 _ _]
      frame #0 {
        n608 = Wait Until Next ms Multiple(millisecond multiple=u32 1000) -> ()  [unwired: 1 out]
        n609 = Divide(x=w1206, y=w1207) -> (x/y=w1205:dbl[])
      }
      frame #1 {
        n610 = Divide(x=w1212, y=w1213) -> (x/y=w1211:dbl[])
      }
      frame #2 {
        n611 = call "Autobalance Initial State DAO.vi"() -> ("Initial Values"=w1217:T1[])  [unwired: 2 in, 9 out]
        n612 = local write "L1 Ctrl Loop State"(Control_Loop_State."Autobalancing" ("L1 Ctrl Loop State")) -> ()
        n613 = Divide(x=w1220, y=w1221) -> (x/y=w1219:dbl[])
      }
      frame #3 {
        n614 = call "Initial Command DAO.vi"("LBCB Number"=w1227, "DAO Actions"=DAO_Actions."Get") -> ("Command Out"=w1229:T36)  [unwired: 2 in, 7 out]
        n615 = call "Actuator Point 2 Array.vi"("Actuator Point"=w1229) -> ("Array"=w1226:dbl[])
        n616 = for {
          tunnel: w1223 -> [w1236] mode=indexing
          tunnel: [w1234] -> w1222 mode=indexing
          n617 = Bundle By Name(cluster=w1236, "IsBalanced"=T2 TRUE) -> (w1234:T1)
        }
        n618 = local write "L1 Ctrl Loop In Actuator"(w1226) -> ()
        n619 = local write "L1 Ctrl Loop State"(Control_Loop_State."Ready for Control" ("L1 Ctrl Loop State")) -> ()
        n620 = Divide(x=w1226, y=w1233) -> (x/y=w1231:dbl[])
        n621 = call "Daq Send.vi"("LBCB Select"=w1227, "Commands"=w1231, "Daq Actions"=Daq_Actions."Send Commands") -> ()  [unwired: 2 in, 7 out]
      }
      frame #4 {
        n622 = local read "L1 Auto Balance Error Tolerance"() -> (w1245:dbl[])
        n623 = local read "L1 Servo Error"() -> (w1239:dbl[])
        n624 = Subtract(x=w1239, y=w1238) -> (x-y=w1240:dbl[])
        n625 = call "Autobalance.vi"("Servo Errors"=w1240, 1:"Autobalance State In"=w1250, "LBCB Number"=w1251, "InitialPosition? In"=w1248, "Error Tolerance"=w1245, "Command In"=w1244, 11:"Autobalance State In"=w1243, "Autobalance \nControl Parameters"=w1237) -> ("IsBalanced"=w1241:T2, "Command Out"=w1246:dbl[], "InitialPosition? Out"=w1247:T2, 14:"Autobalance State Out"=w1249:T26, 15:"Autobalance State Out"=w1242:T1[])  [unwired: 3 out]
        n626 = Multiply(x=w1252, y=w1246) -> (x*y=w1253:dbl[])
        n627 = case shown="True" w1241 {
          tunnel: w1253 -> [_ w1258]
          tunnel: w1251 -> [_ w1256]
          frame #0 {
          }
          frame #1 {
            n628 = call "Array 2 Actuator Point.vi"("Array"=w1258) -> ("Actuator Point"=w1259:T36)
            n629 = call "Initial Command DAO.vi"("Command In"=w1259, "LBCB Number"=w1256, "DAO Actions"=DAO_Actions."Set") -> ()  [unwired: 1 in, 8 out]
            n630 = local write "L1 Ctrl Loop State"(Control_Loop_State."Set Command" ("L1 Ctrl Loop State")) -> ()
          }
        }
        n631 = call "Daq Send.vi"("LBCB Select"=w1251, "Commands"=w1246, "Daq Actions"=Daq_Actions."Send Commands") -> ()  [unwired: 2 in, 7 out]
      }
      frame #5 {
        n632 = Divide(x=w1263, y=w1264) -> (x/y=w1262:dbl[])
      }
      frame #6 {
        # "4. Actiator and Cartesian Limit Check"
        # "3. Actuator to Cartesian, Cartesian to Actuator Conversions"
        n633 = local read "L1 Actuator Meas. Disp & Forces"() -> (w1280:dbl[])
        n634 = local read "L1 Faults"() -> (w1274:T14)
        n635 = Divide(x=w1283, y=1000.0) -> (x/y=w1285:dbl)
        n636 = local read "L1 PID On"() -> (w1279:bool)
        n637 = call "Fault Matrix 2 Bit.vi"("Within Limits"=w1274) -> ("No Faults"=w1273:bool)  [unwired: 10 out]
        n638 = Delete From Array(array=w1280, length=6, index=0) -> (array with subset deleted=w1277:dbl[])  [unwired: 1 out]
        n639 = Select(t=w1269, s=w1273, f=w1268) -> (s? t:f=w1272:dbl[])
        n640 = case shown="False" w1279 {
          tunnel: [w1287 w1293] -> w1271
          tunnel: w1277 -> [_ w1292]
          tunnel: w1272 -> [w1289 w1290]
          tunnel: w1285 -> [_ w1291]
          frame #0 {
            n641 = local read "L1 I Const"() -> (w1288:dbl[])
            n642 = Add(x=w1289, y=w1288) -> (x+y=w1287:dbl[])
          }
          frame #1 {
            n643 = Subtract(x=w1290, y=w1292) -> (x-y=w1298:dbl[])
            n644 = local read "L1 I Gain"() -> (w1299:dbl[])
            n645 = local read "L1 P Gain"() -> (w1294:dbl[])
            n646 = local read "L1 I Const"() -> (w1295:dbl[])
            n647 = Multiply(x=w1298, y=w1294) -> (x*y=w1296:dbl[])
            n648 = Compound Arithmetic op=MULTIPLY(w1298, w1299, w1291) -> (w1300:dbl[])
            n649 = Add(x=w1300, y=w1295) -> (x+y=w1297:dbl[])
            n650 = Compound Arithmetic op=ADD(w1290, w1296, w1297) -> (w1293:dbl[])
            n651 = local write "L1 I Const"(w1297) -> ()
          }
        }
        n652 = Divide(x=w1271, y=w1282) -> (x/y=w1278:dbl[])
        n653 = call "Daq Send.vi"("LBCB Select"=w1281, "Commands"=w1278, "Daq Actions"=Daq_Actions."Send Commands") -> ()  [unwired: 2 in, 7 out]
      }
    }
    n654 = local write "L1 Ctrl Loop Out Actuator"(w1195) -> ()
    n655 = local write "L1 Autobalance Out"(w1190) -> ()
    n656 = local write "L1 Cmd  Volts"(w1185) -> ()
    n657 = Wait Until Next ms Multiple(millisecond multiple=u32 6) -> ()  [unwired: 1 out]
  }
  n658 = local write "L1 Ctrl Loop In Actuator"(w41) -> ()
  n659 = while {
    tunnel: [w1310] -> _
    shift-right: [w1315] -> _
    shift-left: w42 -> [w1318]
    tunnel: w21 -> [w1317]
    shift-right: [w1309] -> _
    shift-left: w56 -> [w1314]
    tunnel: LBCB_Number."LBCB2" ("LBCB Number") -> [w1312]
    tunnel: [w1310] -> w50
    shift-right: [w1308] -> _
    shift-left: _ -> [w1307]
    shift-right: [w1306] -> _
    shift-left: _ -> [w1304]
    shift-right: [w1305] -> _
    shift-left: _ -> [w1303]
    tunnel: w13 -> [_]
    tunnel: w10 -> [w1302]
    tunnel: w6 -> [w1301]
    stop <- w1310 stop-if-true
    # "LBCB 2 Control Loop"
    # "Cartesian\nCommand\nNo  Offset"
    # "Actuator Command"
    n660 = local read "L2 Ctrl Loop In Actuator"() -> (w1316:dbl[])
    n661 = call "GetSamplingRate.vi"() -> ("Sampling"=w1311:i32)
    n662 = local read "App Running"() -> (w1319:bool)
    n663 = local read "L2 Ctrl Loop State"() -> (w1320:T9)
    n664 = local write "L2 Control Rate"(w1311) -> ()
    n665 = Not(x=w1319) -> (.not. x?=w1310:bool)
    n666 = case shown="\"Ready for Control\"" w1320 {
      tunnel: w1311 -> [_ _ _ _ _ _ w1404]
      tunnel: [w1324 w1334 w1341 w1353 w1370 w1384 w1392] -> w1315
      tunnel: w1318 -> [_ w1334 w1341 _ _ w1384 w1389]
      tunnel: w1317 -> [w1325 w1333 w1342 w1358 w1373 w1385 w1403]
      tunnel: w1312 -> [_ _ _ w1348 w1372 _ w1402]
      tunnel: w1316 -> [w1324 _ _ _ _ _ w1390]
      tunnel: [w1326 w1332 w1340 w1355 w1374 w1386 w1398] -> w1308
      tunnel: [w1327 w1335 w1339 w1357 w1366 w1383 w1391] -> w1309
      tunnel: w1314 -> [w1327 w1335 _ w1359 w1367 w1383 w1391]
      tunnel: w1307 -> [_ _ _ w1352 _ _ _]
      tunnel: [w1323 w1331 T2 TRUE ("InitialPosition? Out") w1351 w1369 w1382 w1388] -> w1306
      tunnel: [w1322 w1330 Autobalance_State."Init" ("Autobalance State Out") w1350 w1368 w1381 w1387] -> w1305
      tunnel: w1304 -> [w1323 w1331 _ w1349 w1369 w1382 w1388]
      tunnel: w1303 -> [w1322 w1330 _ w1347 w1368 w1381 w1387]
      tunnel: w1302 -> [_ _ _ w1344 _ _ _]
      tunnel: w1301 -> [_ _ _ w1343 _ _ _]
      frame #0 {
        n667 = Wait Until Next ms Multiple(millisecond multiple=500) -> ()  [unwired: 1 out]
        n668 = Wait Until Next ms Multiple(millisecond multiple=u32 1000) -> ()  [unwired: 1 out]
        n669 = Wait Until Next ms Multiple(millisecond multiple=u32 500) -> ()  [unwired: 1 out]
        n670 = Divide(x=w1324, y=w1325) -> (x/y=w1326:dbl[])
      }
      frame #1 {
        n671 = Divide(x=w1334, y=w1333) -> (x/y=w1332:dbl[])
      }
      frame #2 {
        n672 = local write "L2 Ctrl Loop State"(Control_Loop_State."Autobalancing" ("L1 Ctrl Loop State")) -> ()
        n673 = call "Autobalance Initial State DAO.vi"() -> ("Initial Values"=w1339:T1[])  [unwired: 2 in, 9 out]
        n674 = Divide(x=w1341, y=w1342) -> (x/y=w1340:dbl[])
      }
      frame #3 {
        n675 = local read "L2 Auto Balance Error Tolerance"() -> (w1354:dbl[])
        n676 = local read "L2 Servo Error"() -> (w1346:dbl[])
        n677 = Subtract(x=w1346, y=w1344) -> (x-y=w1345:dbl[])
        n678 = call "Autobalance.vi"("Servo Errors"=w1345, 1:"Autobalance State In"=w1347, "LBCB Number"=w1348, "InitialPosition? In"=w1349, "Error Tolerance"=w1354, "Command In"=w1352, 11:"Autobalance State In"=w1359, "Autobalance \nControl Parameters"=w1343) -> ("IsBalanced"=w1356:T2, "Command Out"=w1355:dbl[], "InitialPosition? Out"=w1351:T2, 14:"Autobalance State Out"=w1350:T26, 15:"Autobalance State Out"=w1357:T1[])  [unwired: 3 out]
        n679 = Multiply(x=w1355, y=w1358) -> (x*y=w1353:dbl[])
        n680 = case shown="True" w1356 {
          tunnel: w1348 -> [_ w1363]
          tunnel: w1353 -> [_ w1362]
          frame #0 {
          }
          frame #1 {
            n681 = call "Array 2 Actuator Point.vi"("Array"=w1362) -> ("Actuator Point"=w1364:T36)
            n682 = local write "L2 Ctrl Loop State"(Control_Loop_State."Set Command" ("L1 Ctrl Loop State")) -> ()
            n683 = call "Initial Command DAO.vi"("Command In"=w1364, "LBCB Number"=w1363, "DAO Actions"=DAO_Actions."Set") -> ()  [unwired: 1 in, 8 out]
          }
        }
        n684 = call "Daq Send.vi"("LBCB Select"=w1348, "Commands"=w1355, "Daq Actions"=Daq_Actions."Send Commands") -> ()  [unwired: 2 in, 7 out]
      }
      frame #4 {
        n685 = call "Initial Command DAO.vi"("LBCB Number"=w1372, "DAO Actions"=DAO_Actions."Get") -> ("Command Out"=w1376:T36)  [unwired: 2 in, 7 out]
        n686 = for {
          tunnel: w1367 -> [w1380] mode=indexing
          tunnel: [w1378] -> w1366 mode=indexing
          n687 = Bundle By Name(cluster=w1380, "IsBalanced"=T2 TRUE) -> (w1378:T1)
        }
        n688 = call "Actuator Point 2 Array.vi"("Actuator Point"=w1376) -> ("Array"=w1370:dbl[])
        n689 = local write "L2 Ctrl Loop In Actuator"(w1370) -> ()
        n690 = local write "L2 Ctrl Loop State"(Control_Loop_State."Ready for Control" ("L1 Ctrl Loop State")) -> ()
        n691 = Divide(x=w1370, y=w1373) -> (x/y=w1374:dbl[])
        n692 = call "Daq Send.vi"("LBCB Select"=w1372, "Commands"=w1374, "Daq Actions"=Daq_Actions."Send Commands") -> ()  [unwired: 2 in, 7 out]
      }
      frame #5 {
        n693 = Divide(x=w1384, y=w1385) -> (x/y=w1386:dbl[])
      }
      frame #6 {
        # "4. Actiator and Cartesian Limit Check"
        # "3. Actuator to Cartesian, Cartesian to Actuator Conversions"
        n694 = local read "L2 Actuator Meas. Disp & Forces"() -> (w1400:dbl[])
        n695 = Divide(x=w1404, y=1000.0) -> (x/y=w1406:dbl)
        n696 = local read "L2 Faults"() -> (w1394:T14)
        n697 = local read "L2 PID On"() -> (w1399:bool)
        n698 = call "Fault Matrix 2 Bit.vi"("Within Limits"=w1394) -> ("No Faults"=w1393:bool)  [unwired: 10 out]
        n699 = Delete From Array(array=w1400, length=6, index=0) -> (array with subset deleted=w1397:dbl[])  [unwired: 1 out]
        n700 = Select(t=w1390, s=w1393, f=w1389) -> (s? t:f=w1401:dbl[])
        n701 = case shown="True" w1399 {
          tunnel: [w1408 w1415] -> w1392
          tunnel: w1397 -> [_ w1414]
          tunnel: w1401 -> [w1410 w1412]
          tunnel: w1406 -> [_ w1413]
          frame #0 {
            n702 = local read "L2 I Const"() -> (w1409:dbl[])
            n703 = Add(x=w1410, y=w1409) -> (x+y=w1408:dbl[])
          }
          frame #1 {
            n704 = local read "L2 I Gain"() -> (w1411:dbl[])
            n705 = Subtract(x=w1412, y=w1414) -> (x-y=w1420:dbl[])
            n706 = local read "L2 P Gain"() -> (w1416:dbl[])
            n707 = local read "L2 I Const"() -> (w1417:dbl[])
            n708 = Multiply(x=w1420, y=w1416) -> (x*y=w1418:dbl[])
            n709 = Compound Arithmetic op=MULTIPLY(w1420, w1411, w1413) -> (w1421:dbl[])
            n710 = Add(x=w1421, y=w1417) -> (x+y=w1419:dbl[])
            n711 = Compound Arithmetic op=ADD(w1412, w1418, w1419) -> (w1415:dbl[])
            n712 = local write "L2 I Const"(w1419) -> ()
          }
        }
        n713 = Divide(x=w1392, y=w1403) -> (x/y=w1398:dbl[])
        n714 = call "Daq Send.vi"("LBCB Select"=w1402, "Commands"=w1398, "Daq Actions"=Daq_Actions."Send Commands") -> ()  [unwired: 2 in, 7 out]
      }
    }
    n715 = local write "L2 Ctrl Loop Out Actuator"(w1315) -> ()
    n716 = local write "L2 Cmd  Volts"(w1308) -> ()
    n717 = local write "L2 Autobalance Out"(w1309) -> ()
    n718 = Wait Until Next ms Multiple(millisecond multiple=u32 6) -> ()  [unwired: 1 out]
  }
  n719 = flat-sequence {
    tunnel: [w1429] -> w26
    tunnel: [w1431] -> w25
    tunnel: [w1430] -> w24
    tunnel: w14 -> [_]
    tunnel: [w1424] -> w11
    tunnel: [w1422] -> w7
    frame #0 {
      n720 = global read "Global Cache.vi" "Autobalance \nControl Parameters"() -> (w1422:T47)
      n721 = global read "Global Cache.vi" "L1 Calibrations"() -> (w1423:T46)
      n722 = Unbundle By Name(w1423) -> ("Command Sensitivity"=w1429:dbl[], "Servo Error Offset"=w1424:dbl[], "LVDT Sensitivity"=w1425:dbl[], "LVDT Offset"=w1428:dbl[], "Load Cell Offsets"=w1427:dbl[], "Load Cell Sensitivity"=w1426:dbl[])
      n723 = Build Array (concatenate)(w1428, w1427) -> (w1431:dbl[])
      n724 = Build Array (concatenate)(w1425, w1426) -> (w1430:dbl[])
    }
  }
  n725 = while {
    shift-right: [w1436] -> _
    shift-left: _ -> [w1443]
    shift-right: [w1437] -> _
    shift-left: w15 -> [w1439]
    tunnel: w59 -> [w1435]
    tunnel: [w1434] -> w44
    stop <- w1434 stop-if-true
    n726 = local read "L1 Ctrl Loop In Actuator"() -> (w1432:dbl[])
    n727 = local read "L2 Ctrl Loop In Actuator"() -> (w1433:dbl[])
    n728 = Build Array (concatenate)(w1432, w1433) -> (w1436:dbl[])
    n729 = Not Equal?(x=w1436, y=w1443) -> (x != y?=w1442:bool[])
    n730 = Or Array Elements(Boolean array=w1442) -> (logical OR=w1441:bool)
    n731 = case shown="False" w1441 {
      tunnel: w1436 -> [_ w1453]
      tunnel: w1439 -> [w1445 w1449]
      tunnel: [w1445 w1447] -> w1438
      tunnel: w1435 -> [_ w1446]
      frame #0 {
      }
      frame #1 {
        n732 = local read "Logging Directory"() -> (w1456:path)
        n733 = Build Path(base path=w1456, name or relative path=w1446) -> (appended path=w1455:path)
        n734 = Open/Create/Replace File(file path (use dialog)=w1455, error in=w1449, operation (0:open)=T58."replace or create") -> (refnum out=w1452:refnum<file>, error out=w1448:errorcluster)  [unwired: 4 out]
        n735 = Write to Binary File(file (use dialog)=w1452, data=w1453, error in=w1448) -> (refnum out=w1450:refnum<file>, error out=w1451:errorcluster)  [unwired: 4 out]
        n736 = Close File(refnum=w1450, error in=w1451) -> (error out=w1447:errorcluster)  [unwired: 1 out]
      }
    }
    n737 = local read "App Running"() -> (w1444:bool)
    n738 = Wait Until Next ms Multiple(millisecond multiple=u32 2000) -> ()  [unwired: 1 out]
    n739 = call "Error Logger.vi"("error in (no error)"=w1438) -> ("error out"=w1437:errorcluster)  [unwired: 1 in, 9 out]
    n740 = Not(x=w1444) -> (.not. x?=w1434:bool)
  }
  n741 = while {
    shift-right: [w1475] -> _
    shift-left: w14 -> [w1480]
    tunnel: w25 -> [w1479]
    tunnel: w24 -> [w1478]
    tunnel: w19 -> [w1474]
    tunnel: w20 -> [w1473]
    tunnel: [w1465] -> w52
    tunnel: w4 -> [w1462]
    shift-right: [w1459] -> _
    shift-left: w2 -> [w1461]
    tunnel: w3 -> [w1460]
    shift-right: [w1458] -> _
    shift-left: FALSE -> [w1457]
    stop <- w1465 stop-if-true
    # "DAQ Loop"
    n742 = local read "DAQ Enabled"() -> (w1477:bool)
    n743 = case shown="True" w1477 {
      tunnel: w1480 -> [w1489 w1516]
      tunnel: [w1489 w1512] -> w1475
      tunnel: w1479 -> [_ w1515]
      tunnel: w1478 -> [_ w1514]
      tunnel: w1474 -> [_ w1511]
      tunnel: w1473 -> [_ w1510]
      tunnel: [w1486 w1508] -> w1471
      tunnel: [w1483 w1507] -> w1470
      tunnel: [w1486 w1506] -> w1469
      tunnel: [w1486 w1505] -> w1468
      tunnel: [w1483 w1504] -> w1467
      tunnel: [_ TRUE] -> w1466
      tunnel: [w1483 w1501] -> w1464
      tunnel: [w1483 w1500] -> w1463
      tunnel: w1462 -> [_ w1498]
      tunnel: w1461 -> [w1481 w1497]
      tunnel: w1460 -> [_ w1496]
      tunnel: [w1481 w1495] -> w1459
      tunnel: [w1482 w1492] -> w1458
      tunnel: w1457 -> [w1482 w1491]
      frame #0 {
        n744 = Initialize Array(0.0 ("element"), 12 ("dimension size")) -> (w1483:dbl[])
        n745 = Initialize Array(0.0 ("element"), 6 ("dimension size")) -> (w1486:dbl[])
        n746 = Wait Until Next ms Multiple(millisecond multiple=u32 500) -> ()  [unwired: 1 out]
      }
      frame #1 {
        n747 = local read "Number of \nExternal \nChannels"() -> (w1513:i32)
        n748 = call "Daq Receive.vi"("Daq Actions"=Daq_Actions."Get Responses", "error in (no error)"=w1516) -> ("Responses"=w1502:dbl[], "error out"=w1494:errorcluster)  [unwired: 1 in, 6 out]
        n749 = local write "DAQ Volts"(w1502) -> ()
        n750 = case shown="False" w1491 {
          selector: w1491 -> [_ w1527]
          tunnel: w1497 -> [w1523 w1528]
          tunnel: w1496 -> [w1525 _]
          tunnel: [w1522 w1528] -> w1495
          tunnel: w1494 -> [w1521 w1526]
          tunnel: [w1520 w1526] -> w1493
          tunnel: [TRUE w1527] -> w1492
          frame #0 {
            n751 = Bundle By Name(cluster=w1525, "Command"=Mixed_Mode_Command_Action."Start Acquisition") -> (w1524:T31)
            n752 = Enqueue Element(queue=w1523, element=w1524, error in (no error)=w1521) -> (queue out=w1522:refnum<queue>, error out=w1520:errorcluster)  [unwired: 1 in, 1 out]
          }
          frame #1 {
          }
        }
        n753 = Unbundle By Name(w1494) -> ("status"=w1509:bool)
        n754 = call "Split DAQ Data.vi"("L1 Absolute Offsets"=w1515, "L1 Measured Sensitivities"=w1514, "Number of LBCBs"=w1498, "Responses"=w1502, "L2 Absolute Offsets"=w1510, "L2 Measured Sensitivities"=w1511, "Number of \nExternal \nChannels"=w1513) -> (3:w1505, "Servo Error"=w1508:dbl[][], "LVDT & LC"=w1507:dbl[][], "External Channels"=w1506:dbl[], "Volts LVDT & LC"=w1501:dbl[][], 14:w1504, 15:w1500)  [unwired: 2 out]
        n755 = Wait Until Next ms Multiple(millisecond multiple=u32 6) -> ()  [unwired: 1 out]
        n756 = call <vilib>:"Clear Errors.vi"("error in (no error)"=w1493) -> ("error out"=w1512:errorcluster)  [unwired: 6 out]
        n757 = local write "DAQ Overflow"(w1509) -> ()
      }
    }
    n758 = local write "DAQ Started"(w1466) -> ()
    n759 = local write "L1 Servo Error"(w1471) -> ()
    n760 = local write "External Sensors"(w1469) -> ()
    n761 = local read "App Running"() -> (w1476:bool)
    n762 = local write "L1 Volts LVDT & LC"(w1464) -> ()
    n763 = local write "L2 Volts LVDT & LC"(w1463) -> ()
    n764 = local write "L1 Actuator Meas. Disp & Forces"(w1470) -> ()
    n765 = call "GetSamplingRate.vi"() -> ("Sampling"=w1472:i32)
    n766 = local write "L2 Actuator Meas. Disp & Forces"(w1467) -> ()
    n767 = local write "L2 Servo Error"(w1468) -> ()
    n768 = local write "DAQ Rate"(w1472) -> ()
    n769 = Not(x=w1476) -> (.not. x?=w1465:bool)
  }
  n770 = Obtain Queue(element data type="", error in (no error)=w14) -> (queue out=w32:refnum<queue>, error out=w31:errorcluster)  [unwired: 2 in, 2 out]
  n771 = while {
    shift-right: [w1531] -> _
    shift-left: w32 -> [w1534]
    shift-right: [w1532] -> _
    shift-left: w31 -> [w1533]
    tunnel: [w1529] -> w30
    stop <- w1529 stop-if-true
    # "Archive Voltage Readings"
    n772 = Get Queue Status(queue=w1534, error in (no error)=w1533) -> (queue out=w1537:refnum<queue>, error out=w1538:errorcluster, # elements in queue=w1536:i32)  [unwired: 6 out]
    n773 = Wait Until Next ms Multiple(millisecond multiple=u32 2000) -> ()  [unwired: 1 out]
    n774 = Greater Than 0?(x=w1536) -> (x > 0?=w1535:bool)
    n775 = case shown="False" w1535 {
      tunnel: w1537 -> [w1542 w1551]
      tunnel: w1538 -> [w1541 w1550]
      tunnel: [w1541 w1547] -> w1539
      tunnel: [w1542 w1549] -> w1531
      frame #0 {
        n776 = Wait Until Next ms Multiple(millisecond multiple=u32 100) -> ()  [unwired: 1 out]
      }
      frame #1 {
        n777 = Flush Queue(queue=w1551, error in (no error)=w1550) -> (queue out=w1549:refnum<queue>, remaining elements=w1546:string[], error out=w1548:errorcluster)
        n778 = Concatenate Strings(w1546) -> (w1545:string)
        n779 = call "Save Text Data.vi"("LogFile Type"=LogFileType."Volts", "error in"=w1548, "String"=w1545) -> ("error out"=w1547:errorcluster)  [unwired: 1 in, 1 out]
      }
    }
    n780 = local read "App Running"() -> (w1540:bool)
    n781 = Not(x=w1540) -> (.not. x?=w1529:bool)
    n782 = call "Error Logger.vi"("error in (no error)"=w1539) -> ("error out"=w1532:errorcluster)  [unwired: 1 in, 9 out]
  }
  n783 = while {
    shift-right: [w1554] -> _
    shift-left: w32 -> [w1556]
    shift-right: [w1553] -> _
    shift-left: w31 -> [w1555]
    tunnel: [w1552] -> w29
    stop <- w1552 stop-if-true
    # "Collect Voltage Readings"
    n784 = call "App Status Globals.vi"("App Status Actions"=App_Status_Actions."Get Status") -> ("App Status Out"=w1560:T51)  [unwired: 5 in, 9 out]
    n785 = Unbundle By Name(w1560) -> ("Voltage Logging"=w1558:bool)
    n786 = local read "Volt Logger Time"() -> (w1557:u32)
    n787 = case shown="False" w1558 {
      tunnel: w1556 -> [w1563 w1568]
      tunnel: w1555 -> [w1562 w1567]
      tunnel: [w1563 w1565] -> w1554
      tunnel: [w1562 w1564] -> w1553
      frame #0 {
      }
      frame #1 {
        n788 = local read "L1 Cmd  Volts"() -> (w1572:dbl[])
        n789 = local read "L2 Cmd  Volts"() -> (w1571:dbl[])
        n790 = local read "DAQ Volts"() -> (w1570:dbl[])
        n791 = Build Array (concatenate)(w1572, w1571, w1570) -> (w1569:dbl[])
        n792 = call "Data 2 Record.vi"("Data"=w1569) -> ("Records"=w1566:string)  [unwired: 1 in, 9 out]
        n793 = Enqueue Element(queue=w1568, element=w1566, error in (no error)=w1567) -> (queue out=w1565:refnum<queue>, error out=w1564:errorcluster)  [unwired: 2 out]
      }
    }
    n794 = Wait Until Next ms Multiple(millisecond multiple=w1557) -> ()  [unwired: 1 out]
    n795 = local read "App Running"() -> (w1561:bool)
    n796 = Not(x=w1561) -> (.not. x?=w1552:bool)
  }
  n797 = Obtain Queue(element data type="", error in (no error)=w14) -> (queue out=w55:refnum<queue>, error out=w28:errorcluster)  [unwired: 2 in, 2 out]
  n798 = while {
    shift-right: [w1578] -> _
    shift-left: w55 -> [w1584]
    shift-right: [w1576] -> _
    shift-left: w14 -> [w1581]
    tunnel: [w1574] -> w45
    stop <- w1574 stop-if-true
    # "Write Mixed Mode State"
    n799 = Get Queue Status(queue=w1584, error in (no error)=w1581) -> (queue out=w1580:refnum<queue>, error out=w1579:errorcluster, # elements in queue=w1582:i32)  [unwired: 6 out]
    n800 = Wait Until Next ms Multiple(millisecond multiple=u32 2000) -> ()  [unwired: 1 out]
    n801 = Greater Than 0?(x=w1582) -> (x > 0?=w1583:bool)
    n802 = case shown="False" w1583 {
      tunnel: w1580 -> [w1586 w1595]
      tunnel: w1579 -> [w1585 w1594]
      tunnel: [w1585 w1591] -> w1577
      tunnel: [w1586 w1593] -> w1578
      frame #0 {
        n803 = Wait Until Next ms Multiple(millisecond multiple=u32 100) -> ()  [unwired: 1 out]
      }
      frame #1 {
        n804 = Flush Queue(queue=w1595, error in (no error)=w1594) -> (queue out=w1593:refnum<queue>, remaining elements=w1590:string[], error out=w1592:errorcluster)
        n805 = Concatenate Strings(w1590) -> (w1589:string)
        n806 = call "Save Text Data.vi"("LogFile Type"=LogFileType."Mixed Mode State", "error in"=w1592, "String"=w1589) -> ("error out"=w1591:errorcluster)  [unwired: 1 in, 1 out]
      }
    }
    n807 = local read "App Running"() -> (w1575:bool)
    n808 = Not(x=w1575) -> (.not. x?=w1574:bool)
    n809 = call "Error Logger.vi"("error in (no error)"=w1577) -> ("error out"=w1576:errorcluster)  [unwired: 1 in, 9 out]
  }
  n810 = while {
    shift-right: [w1611] -> _
    shift-left: w53 -> [w1613]
    shift-right: [w1609] -> _
    shift-left: w28 -> [w1612]
    shift-right: [w1608] -> _
    shift-left: w55 -> [w1606]
    tunnel: [w1603] -> w46
    stop <- w1603 stop-if-true
    # "Collect Mixed Mode State"
    n811 = Wait on Notification(notifier=w1613, timeout in ms (-1)=200, error in (no error)=w1612) -> (notifier out=w1611:refnum<notifier>, notification=w1597:T24, timed out?=w1599:bool, error out=w1605:errorcluster)  [unwired: 1 out]
    n812 = call "App Status Globals.vi"("App Status Actions"=App_Status_Actions."Get Status") -> ("App Status Out"=w1601:T51)  [unwired: 5 in, 9 out]
    n813 = Unbundle By Name(w1601) -> ("Mixed Mode Logging"=w1600:bool)
    n814 = Compound Arithmetic op=AND(w1600, invert w1599) -> (w1598:bool)
    n815 = Select(t=w1597, s=w1598, f=Mixed_Mode_States."Nop" ("t")) -> (s? t:f=w1607:T24)
    n816 = case shown="\"Nop\"" w1607 {
      selector: w1607 -> [w1619 w1623 w1628 w1643 w1669 w1687 _]
      tunnel: w1605 -> [w1616 w1622 w1641 w1656 w1679 w1694 w1697]
      tunnel: [w1615 w1624 w1629 w1644 w1672 w1688 w1697] -> w1610
      tunnel: w1606 -> [w1620 w1626 w1635 w1648 w1676 w1690 w1698]
      tunnel: [w1618 w1625 w1631 w1649 w1677 w1691 w1698] -> w1608
      frame #0 {
        n817 = call "Archive Mixed Mode State.vi"("MixedModeStates"=w1619) -> ("string"=w1617:string)  [unwired: 1 in, 9 out]
        n818 = Enqueue Element(queue=w1620, element=w1617, error in (no error)=w1616) -> (queue out=w1618:refnum<queue>, error out=w1615:errorcluster)  [unwired: 2 out]
      }
      frame #1 {
        n819 = call "Archive Mixed Mode State.vi"("MixedModeStates"=w1623) -> ("string"=w1621:string)  [unwired: 1 in, 9 out]
        n820 = Enqueue Element(queue=w1626, element=w1621, error in (no error)=w1622) -> (queue out=w1625:refnum<queue>, error out=w1624:errorcluster)  [unwired: 2 out]
      }
      frame #2 {
        n821 = local read "L1 Convergence Status"() -> (w1636:T23)
        n822 = local read "L2 Convergence Status"() -> (w1637:T23)
        n823 = call "Archive Mixed Mode State.vi"("MixedModeStates"=w1628) -> ("string"=w1627:string)  [unwired: 1 in, 9 out]
        n824 = call "Archive Convergence Status.vi"("error in"=w1641, "LBCB Filter"=LBCB_Filter."LBCB 1", "Convergence Status"=w1636) -> ("error out"=w1639:errorcluster, "string"=w1634:string)  [unwired: 7 out]
        n825 = call "Archive Convergence Status.vi"("error in"=w1639, "LBCB Filter"=LBCB_Filter."LBCB 2", "Convergence Status"=w1637) -> ("error out"=w1630:errorcluster, "string"=w1633:string)  [unwired: 7 out]
        n826 = Concatenate Strings(w1627, w1634, w1633) -> (w1632:string)
        n827 = Enqueue Element(queue=w1635, element=w1632, error in (no error)=w1630) -> (queue out=w1631:refnum<queue>, error out=w1629:errorcluster)  [unwired: 2 out]
      }
      frame #3 {
        n828 = local read "L1 Convergence Status"() -> (w1651:T23)
        n829 = call "Archive Mixed Mode State.vi"("MixedModeStates"=w1643) -> ("string"=w1642:string)  [unwired: 1 in, 9 out]
        n830 = local read "L2 Convergence Status"() -> (w1652:T23)
        n831 = call "Archive Convergence Status.vi"("error in"=w1656, "LBCB Filter"=LBCB_Filter."LBCB 1", "Convergence Status"=w1651) -> ("error out"=w1654:errorcluster, "string"=w1647:string)  [unwired: 7 out]
        n832 = call "Archive Convergence Status.vi"("error in"=w1654, "LBCB Filter"=LBCB_Filter."LBCB 2", "Convergence Status"=w1652) -> ("error out"=w1645:errorcluster, "string"=w1646:string)  [unwired: 7 out]
        n833 = Concatenate Strings(w1642, w1647, w1646) -> (w1650:string)
        n834 = Enqueue Element(queue=w1648, element=w1650, error in (no error)=w1645) -> (queue out=w1649:refnum<queue>, error out=w1644:errorcluster)  [unwired: 2 out]
      }
      frame #4 {
        w1663 = "Previous" ("Prefix")
        w1665 = "Current" ("Prefix")
        w1661 = LBCB_Number."LBCB2" ("LBCB Number")
        w1662 = LBCB_Number."LBCB1" ("LBCB Number")
        n835 = local read "L2 Stiffness Jacobian"() -> (w1680:T22)
        n836 = local read "L2 Measurements"() -> (w1666:T21)
        n837 = local read "L1 Measurements"() -> (w1668:T21)
        n838 = local read "L1 Previous Target"() -> (w1667:T5)
        n839 = local read "L2 Previous Target"() -> (w1664:T5)
        n840 = local read "L1 Stiffness Jacobian"() -> (w1681:T22)
        n841 = call "Archive Mixed Mode State.vi"("MixedModeStates"=w1669) -> ("string"=w1670:string)  [unwired: 1 in, 9 out]
        n842 = call "Archive Measurement Data.vi"("Prefix"=w1665, "LBCB Number"=w1662, "Data"=w1668) -> ("string"=w1660:string)  [unwired: 1 in, 7 out]
        n843 = call "Archive Target Data.vi"("Prefix"=w1663, "LBCB Number"=w1662, "Data"=w1667) -> ("string"=w1659:string)  [unwired: 1 in, 7 out]
        n844 = call "Archive Stiffness Jacobian.vi"("error in (no error)"=w1679, "LBCB Number"=w1662, "LBCB  Stiffness Jacobian"=w1681) -> ("error out"=w1678:errorcluster, "String"=w1675:string)  [unwired: 7 out]
        n845 = call "Archive Measurement Data.vi"("Prefix"=w1665, "LBCB Number"=w1661, "Data"=w1666) -> ("string"=w1658:string)  [unwired: 1 in, 7 out]
        n846 = call "Archive Stiffness Jacobian.vi"("error in (no error)"=w1678, "LBCB Number"=w1661, "LBCB  Stiffness Jacobian"=w1680) -> ("error out"=w1673:errorcluster, "String"=w1674:string)  [unwired: 7 out]
        n847 = call "Archive Target Data.vi"("Prefix"=w1663, "LBCB Number"=w1661, "Data"=w1664) -> ("string"=w1657:string)  [unwired: 1 in, 7 out]
        n848 = Concatenate Strings(w1670, w1675, w1674, w1660, w1659, w1658, w1657) -> (w1671:string)
        n849 = Enqueue Element(queue=w1676, element=w1671, error in (no error)=w1673) -> (queue out=w1677:refnum<queue>, error out=w1672:errorcluster)  [unwired: 2 out]
      }
      frame #5 {
        n850 = local read "L2 Iterative Target"() -> (w1696:T6)
        n851 = local read "L1 Iterative Target"() -> (w1695:T6)
        n852 = call "Archive Mixed Mode State.vi"("MixedModeStates"=w1687) -> ("string"=w1686:string)  [unwired: 1 in, 9 out]
        n853 = call "Archive Command Data.vi"("error in"=w1694, "LBCB Filter"=LBCB_Filter."LBCB 1", "Command Data"=w1695) -> ("error out"=w1693:errorcluster, "string"=w1683:string)  [unwired: 7 out]
        n854 = call "Archive Command Data.vi"("error in"=w1693, "LBCB Filter"=LBCB_Filter."LBCB 2", "Command Data"=w1696) -> ("error out"=w1689:errorcluster, "string"=w1682:string)  [unwired: 7 out]
        n855 = Concatenate Strings(w1686, w1683, w1682) -> (w1692:string)
        n856 = Enqueue Element(queue=w1690, element=w1692, error in (no error)=w1689) -> (queue out=w1691:refnum<queue>, error out=w1688:errorcluster)  [unwired: 2 out]
      }
      frame #6 {
      }
    }
    n857 = local read "App Running"() -> (w1604:bool)
    n858 = Not(x=w1604) -> (.not. x?=w1603:bool)
    n859 = call "Error Logger.vi"("error in (no error)"=w1610) -> ("error out"=w1609:errorcluster)  [unwired: 1 in, 9 out]
  }
  n860 = Compound Arithmetic op=AND(w44, w52, w51, w50, w49, w48, w47, w46, w45, w30, w29) -> (w43:bool)
  n861 = flat-sequence {
    tunnel: w43 -> [w1701]
    frame #0 {
      n862 = local write "All Stopped"(w1701) -> ()
      n863 = call "NoArgumentsLauncher.vi"("Application"=NoPanelAppTypes."Control Loops", "Application Launcher Actions"=Launcher_Actions."Stop") -> ()  [unwired: 1 in, 9 out]
    }
  }
